vi "Autonomous Independent.vi"() -> ()   [LabVIEW 2023]
doc: "This VI is called when autonomous begins, and will automatically be terminated when autonomous ends. You can carry out timed or sensor driven robot movement independently without needing to return to the caller."
uses:
  <vilib>/Rock Robotics/WPI/ThirdParty/Phoenix-LabVIEW/Motor Controller/Controls/CTRE_Phoenix_MotorControl_ControlMode.ctl
  <vilib>/Rock Robotics/WPI/Utilities/WPI_GetSetVariantRefNum.vi
  <vilib>/Rock Robotics/Network Tables/NT Read String.vi
  <vilib>/Rock Robotics/Network Tables/NT Write Numeric Array.vi
  <vilib>/Rock Robotics/WPI/ThirdParty/Phoenix-LabVIEW/Motor Controller/Get/CTRE_Phoenix_MotorController_GetSelectedSensorData.vi
  <vilib>/Rock Robotics/WPI/ThirdParty/Phoenix-LabVIEW/Pigeon IMU/CTRE_PigeonIMU_GetAccumGyro.vi
  <vilib>/Rock Robotics/WPI/RobotDrive/WPI_RobotDriveArcadeDrive_Standard(NoSaturation).vi
panel:
  out "Limit Switch":bool=TRUE
  out "Y":dbl
  out "X":dbl
  out "Z":dbl
  out "Talon FX LEFT Moter Encoders":i32
  out "Current Movement, for debugging":T1 {"Y Joystick Value" scale=1.0..-1.0; "X Joystick Value" scale=-1.0..1.0}
  in  "Array of robot movements":T2(array[cluster])=[{"X Joystick Value"=0.39393939393939403, "Y Joystick Value"=0.0, "Delay (sec)"=1.0, "Movement Name"="turn"}, {"X Joystick Value"=-0.3737373737373737, "Y Joystick Value"=0.0, "Delay (sec)"=1.0, "Movement Name"="turn back"}] {"Y Joystick Value" scale=1.0..-1.0; "X Joystick Value" scale=-1.0..1.0}
  # "Be sure to right-click and choose Data Operations>>Make Current Value default if you want to save the array values with the VI"
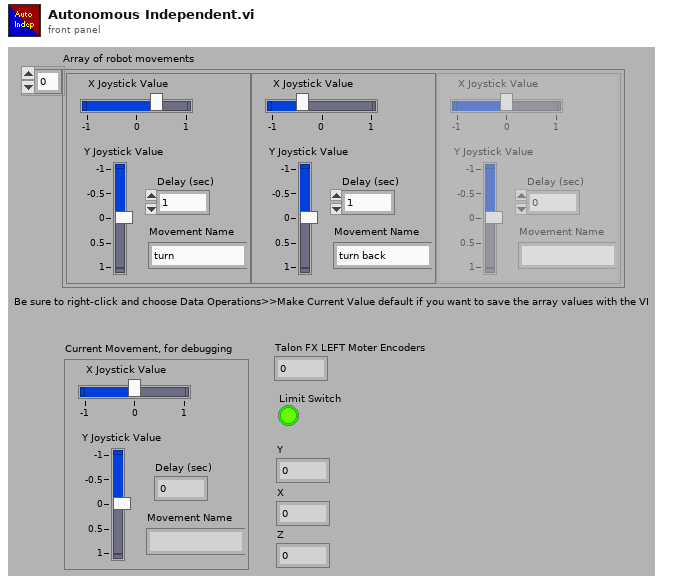
[diagram p1: front panel]
types:
  T1 = cluster{"X Joystick Value":dbl, "Y Joystick Value":dbl, "Delay (sec)":dbl, "Movement Name":string}
  T2 = cluster{"X Joystick Value":dbl, "Y Joystick Value":dbl, "Delay (sec)":dbl, "Movement Name":string}[]
  T3 = typedef "WPI_JoystickDevRef.ctl" = cluster{"Device":T4}
  T4 = typedef "WPI_JoystickDeviceEnum.ctl" = enum16{"USB 0", "USB 1", "USB 2", "USB 3", "USB 4", "USB 5"}
  T5 = typedef "WPI_RobotDriveDevRef.ctl" = cluster{"DevStatus":errorcluster, "Motors[]":T6[], "Square Inputs":bool, "Max Output":dbl}
  T6 = typedef "WPI_MotorControlDeviceRef.ctl" = cluster{"DeviceStatus":errorcluster, "Type":T7, "PWM":cluster{"PWM Channel":T8, "DeadBand":T9}, "CAN":cluster{"Device Number":u8, "SetOutput VI Ref":variant, "GetOutput VI Ref":variant, "Enable VI Ref":variant, "Disable VI Ref":variant, "Data":variant}, "Invert":bool, "DIO PWM":cluster{"PWM \"Enable\" Channel":T8, "DIOChannel":T10, "PWM Rate":dbl}}
  T7 = typedef "WPI_MotorControlType.ctl" = enum16{"PWM", "CAN", "DIO PWM"}
  T8 = typedef "FPGA_DIOPWMChannel.ctl" = enum8{"PWM 0", "PWM 1", "PWM 2", "PWM 3", "PWM 4", "PWM 5", "PWM 6", "PWM 7", "PWM 8", "PWM 9", "PWM MXP 0", "PWM MXP 1", "PWM MXP 2", "PWM MXP 3", "PWM MXP 4", "PWM MXP 5", "PWM MXP 6", "PWM MXP 7", "PWM MXP 8", "PWM MXP 9", "Invalid"}
  T9 = typedef "WPI_PWMDeadband.ctl" = cluster{"Name":string, "maxPositivePwm":i32, "minPositivePwm":i32, "centerPwm":i32, "maxNegativePwm":i32, "minNegativePwm":i32, "angularRange":u16}
  T10 = typedef "FPGA_DIOChannel.ctl" = enum8{"DIO 0", "DIO 1", "DIO 2", "DIO 3", "DIO 4", "DIO 5", "DIO 6", "DIO 7", "DIO 8", "DIO 9", "DIO MXP 0", "DIO MXP 1", "DIO MXP 2", "DIO MXP 3", "DIO MXP 4", "DIO MXP 5", "DIO MXP 6", "DIO MXP 7", "DIO MXP 8", "DIO MXP 9", "DIO MXP 10", "DIO MXP 11", "DIO MXP 12", "DIO MXP 13", "DIO MXP 14", "DIO MXP 15", "SPI Port CS1", "SPI Port CS2", "SPI Port CS3", "SPI Port MISO", "SPI Port MOSI", "Invalid"}
  T11 = typedef "CTRE_Phoenix_MotorControl_ControlMode.ctl" = u16
  T12 = typedef "CTRE_PigeonIMU_DeviceRef.ctl" = cluster{"DeviceStatus":errorcluster, "Device Number":u8, "Type":T13, "Device ID":u32, "Handle":u64, "UsageFrame":u32, "Library Path":path}
  T13 = typedef "CTRE_PigeonIMU_ConnectionType.ctl" = u32
  T14 = typedef "WPI_SwitchDevRef.ctl" = cluster{"DevStatus":errorcluster, "DIO Channel":T10, "CntIndex":T15, "Normally Closed":bool}
  T15 = typedef "FPGA_CounterCtrSystemIndex.ctl" = enum8{"Ctr 0", "Ctr 1", "Ctr 2", "Ctr 3", "Ctr 4", "Ctr 5", "Ctr 6", "Ctr 7", "Invalid"}
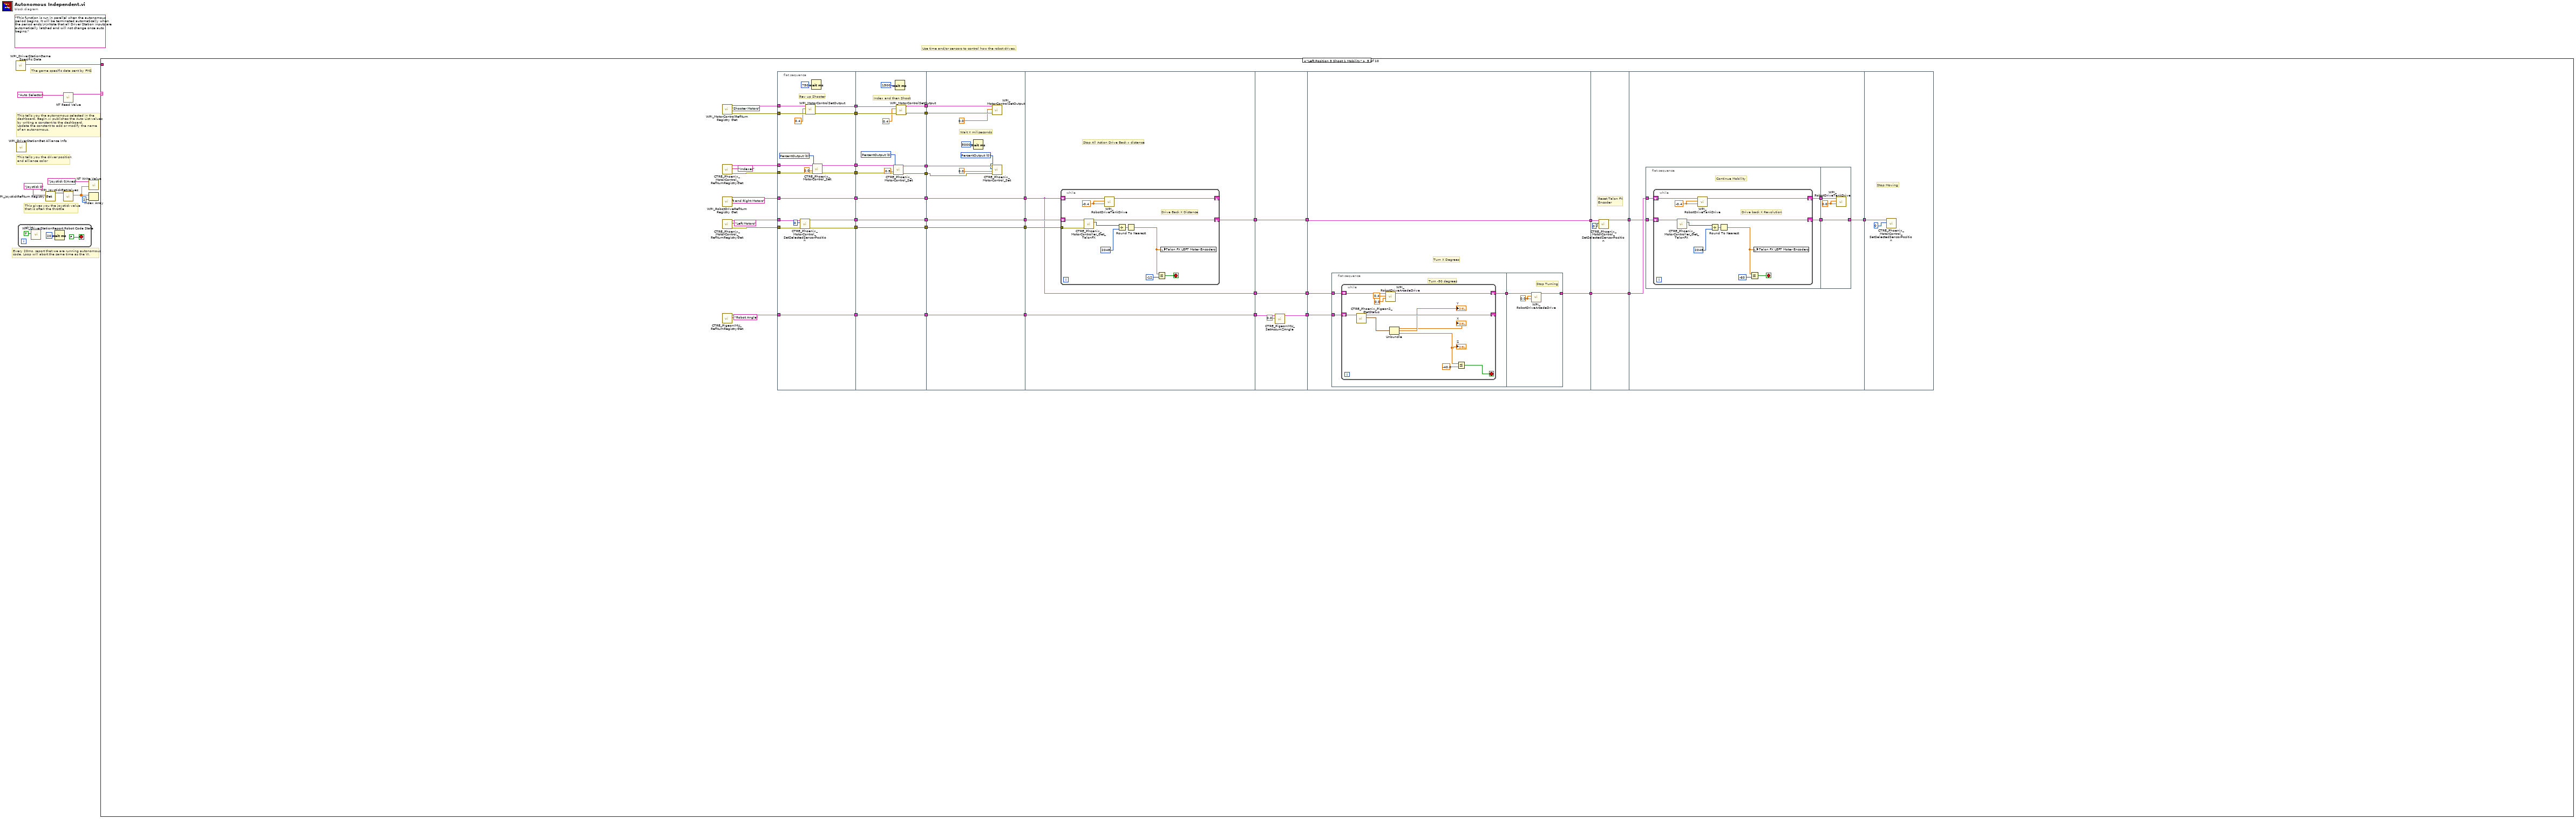
[diagram p0: block diagram]
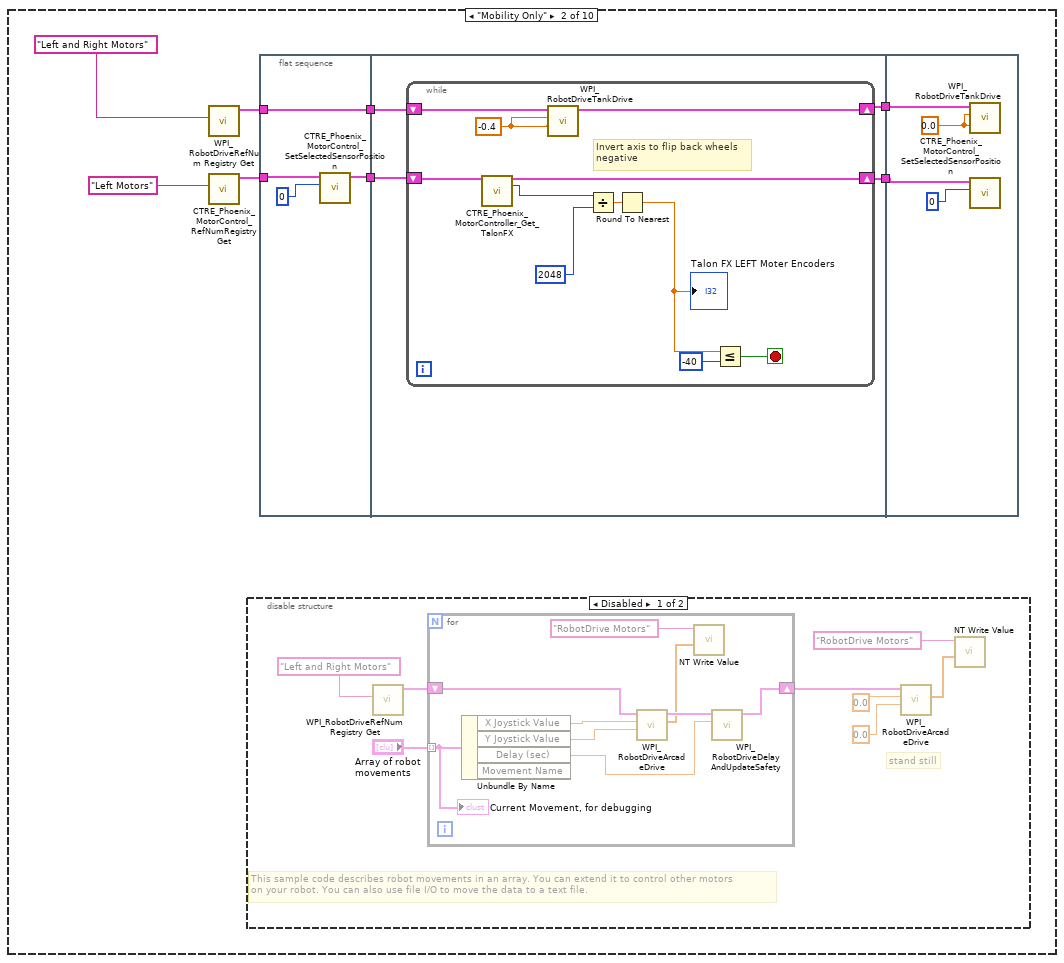
[diagram p3: hidden frame]
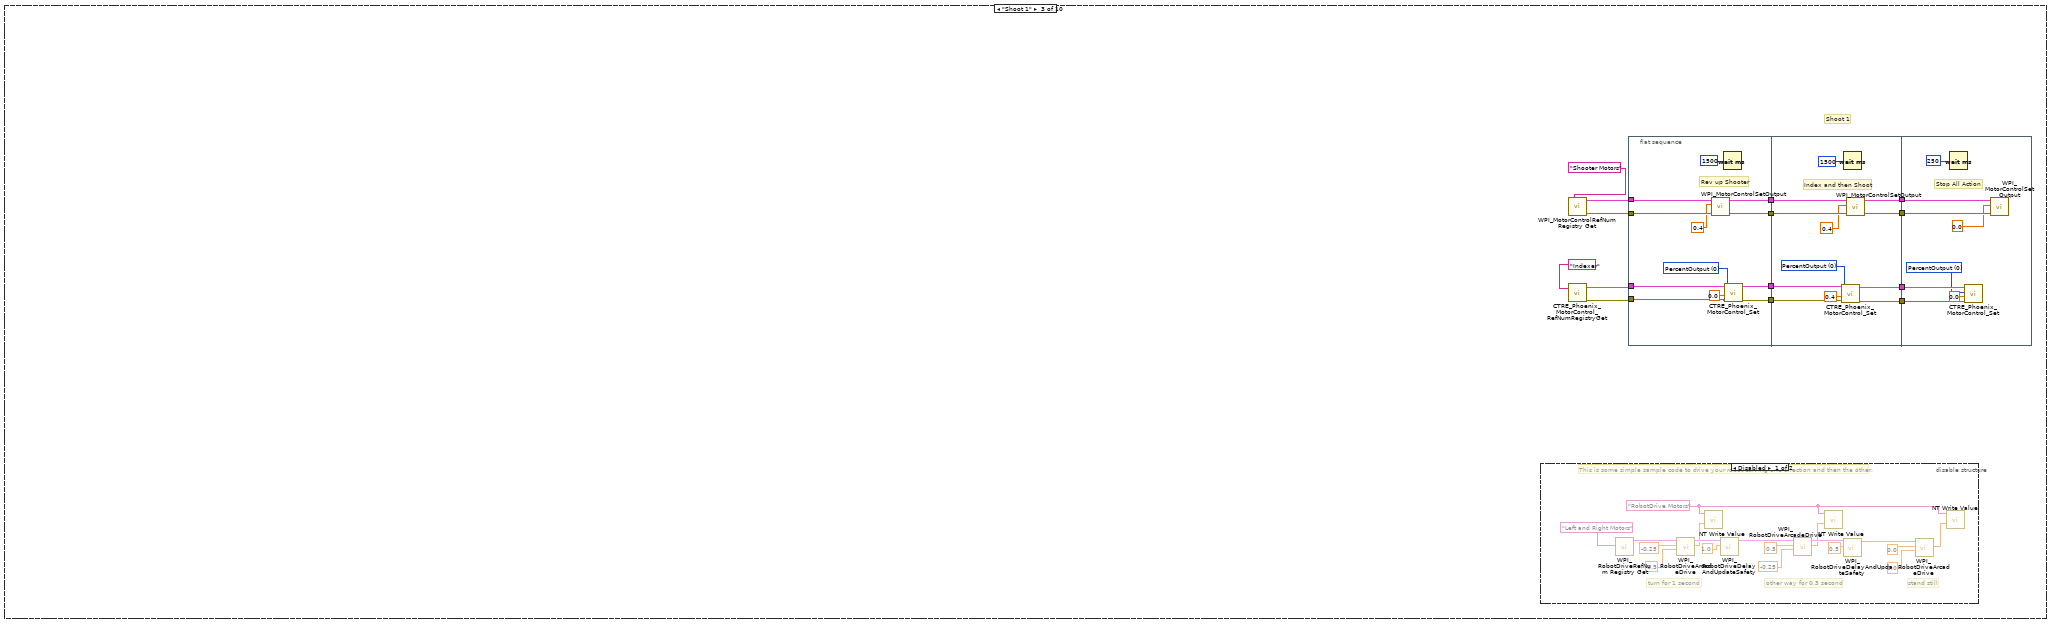
[diagram p5: hidden frame]
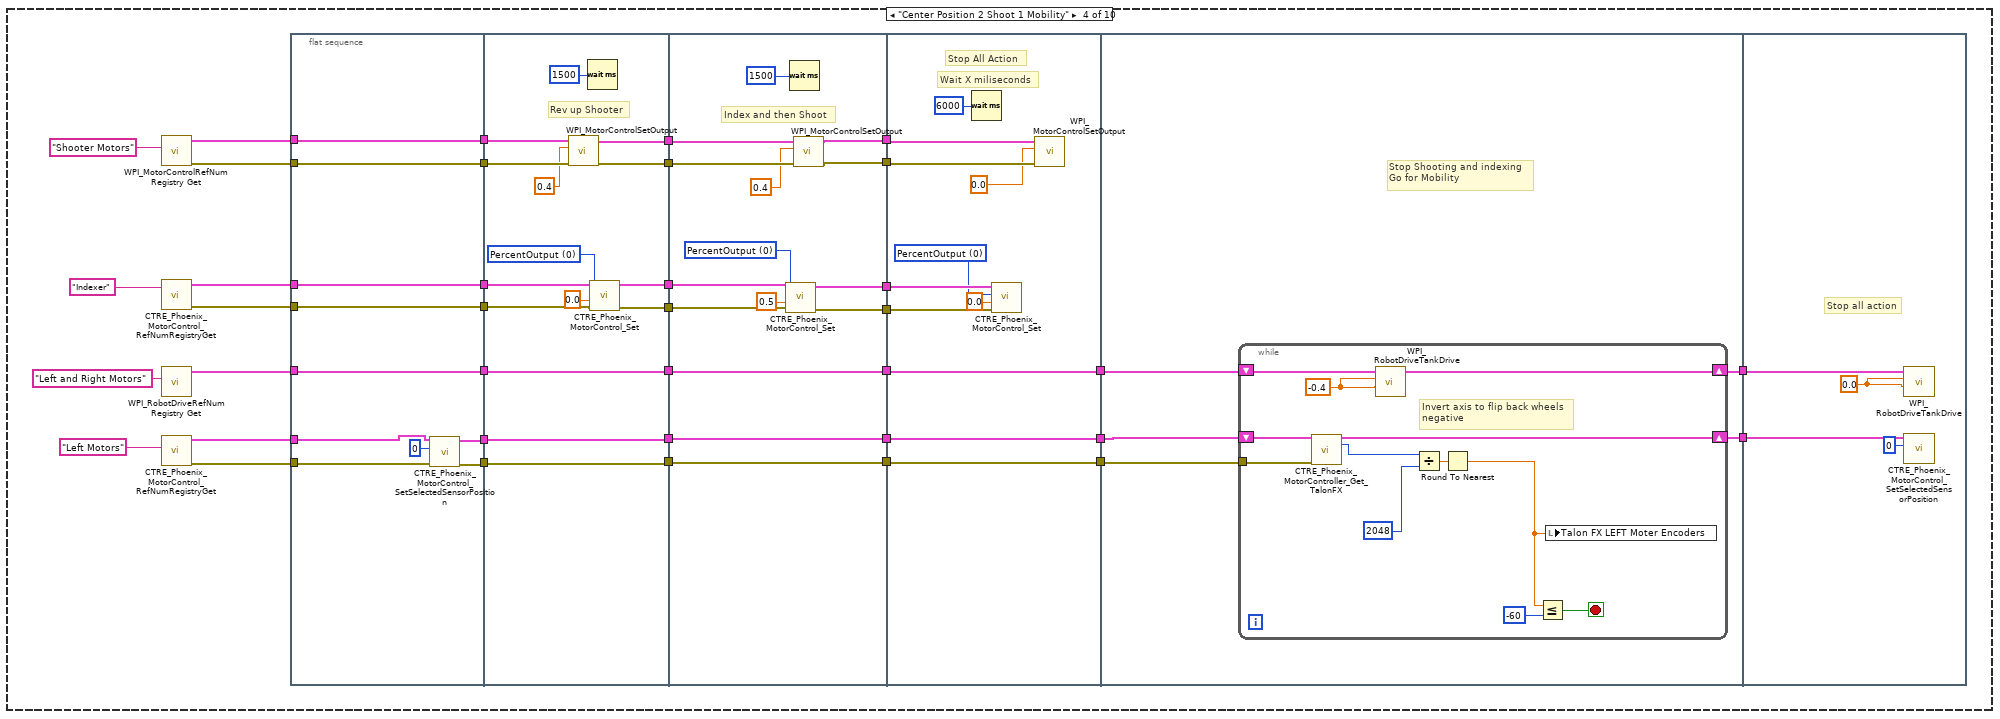
[diagram p7: hidden frame]
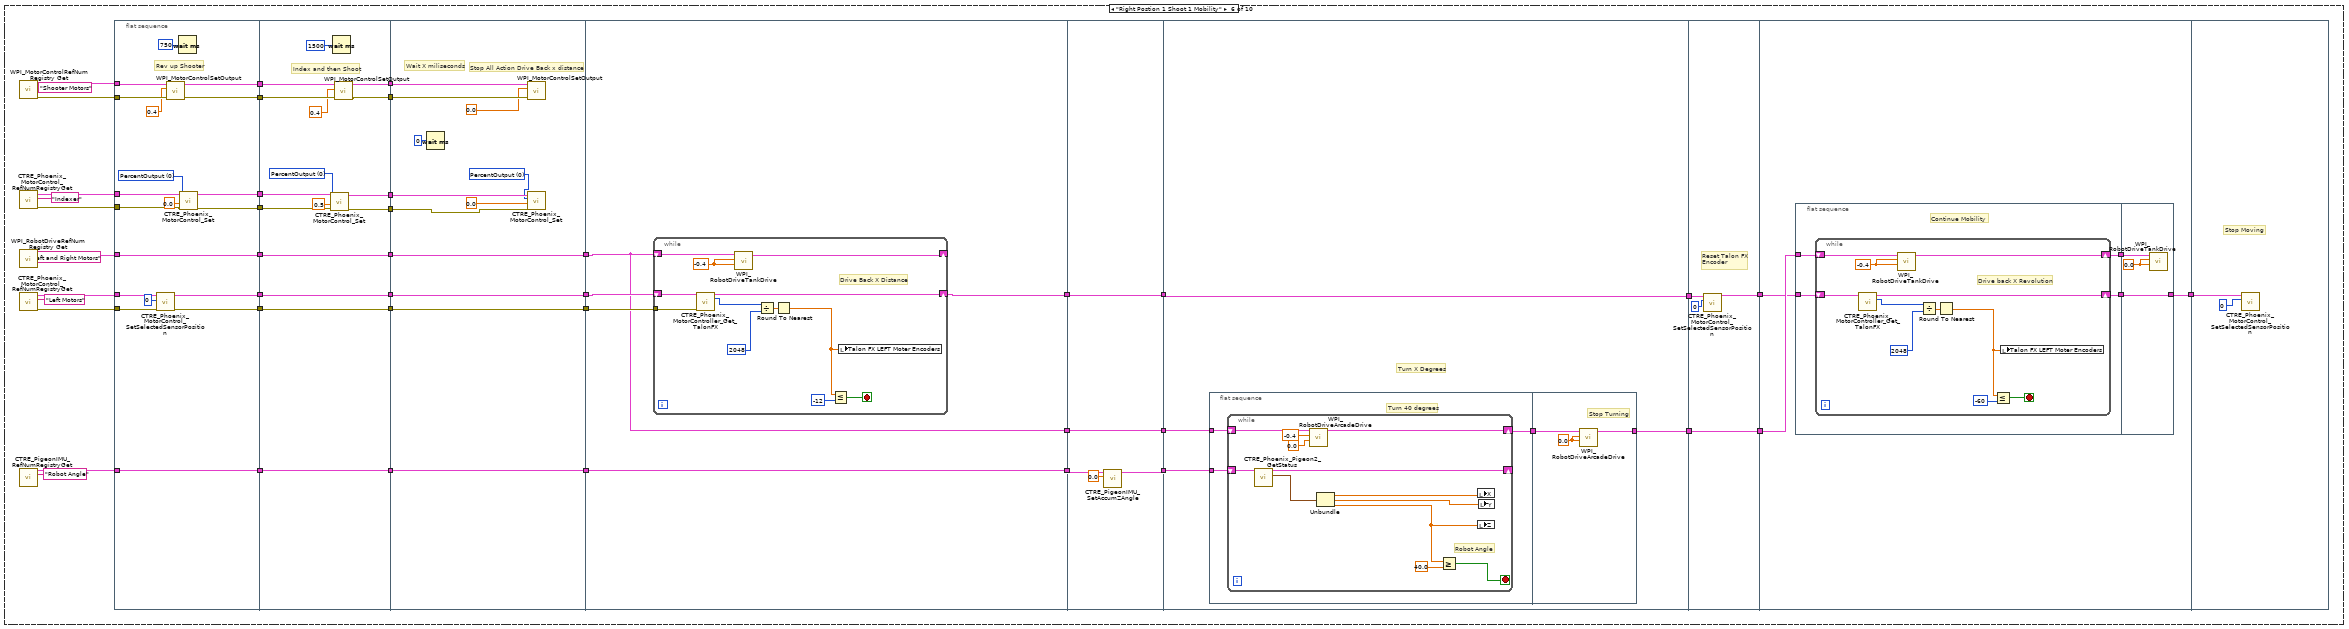
[diagram p8: hidden frame]
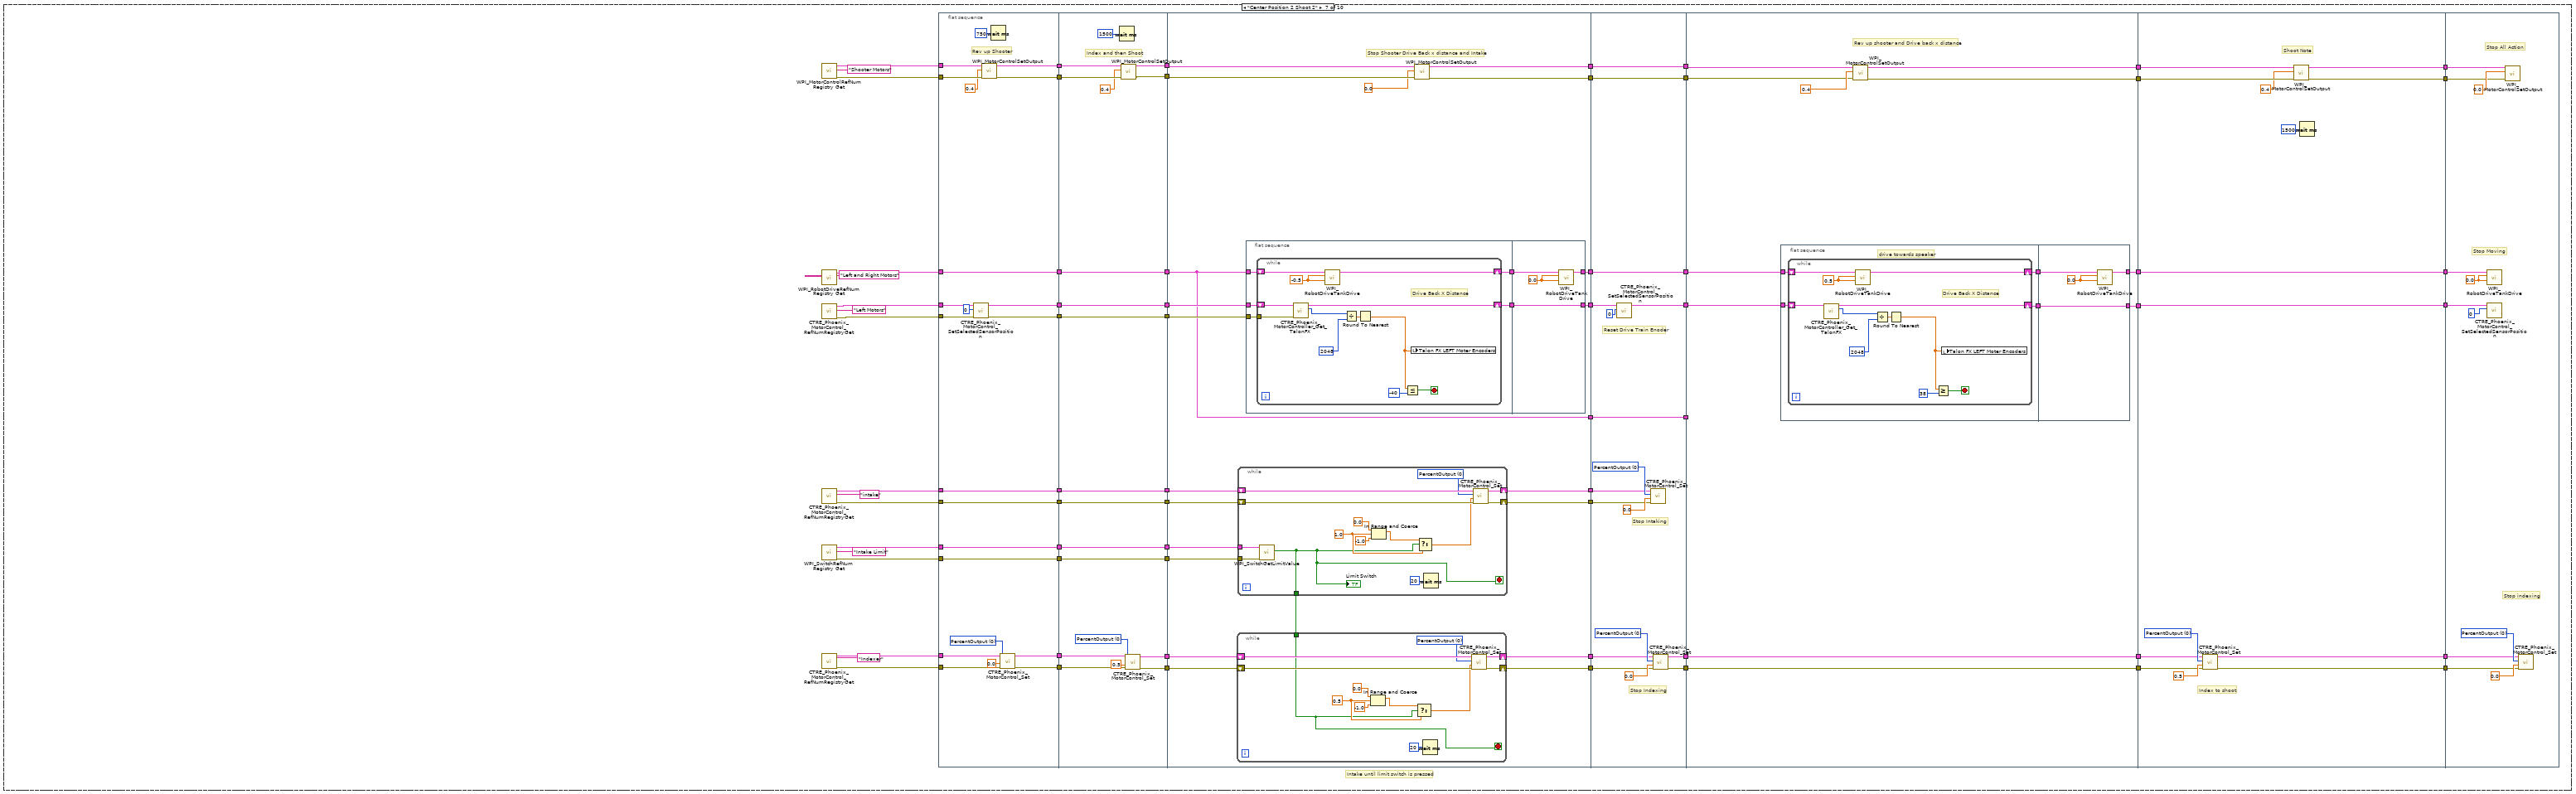
[diagram p9: hidden frame]
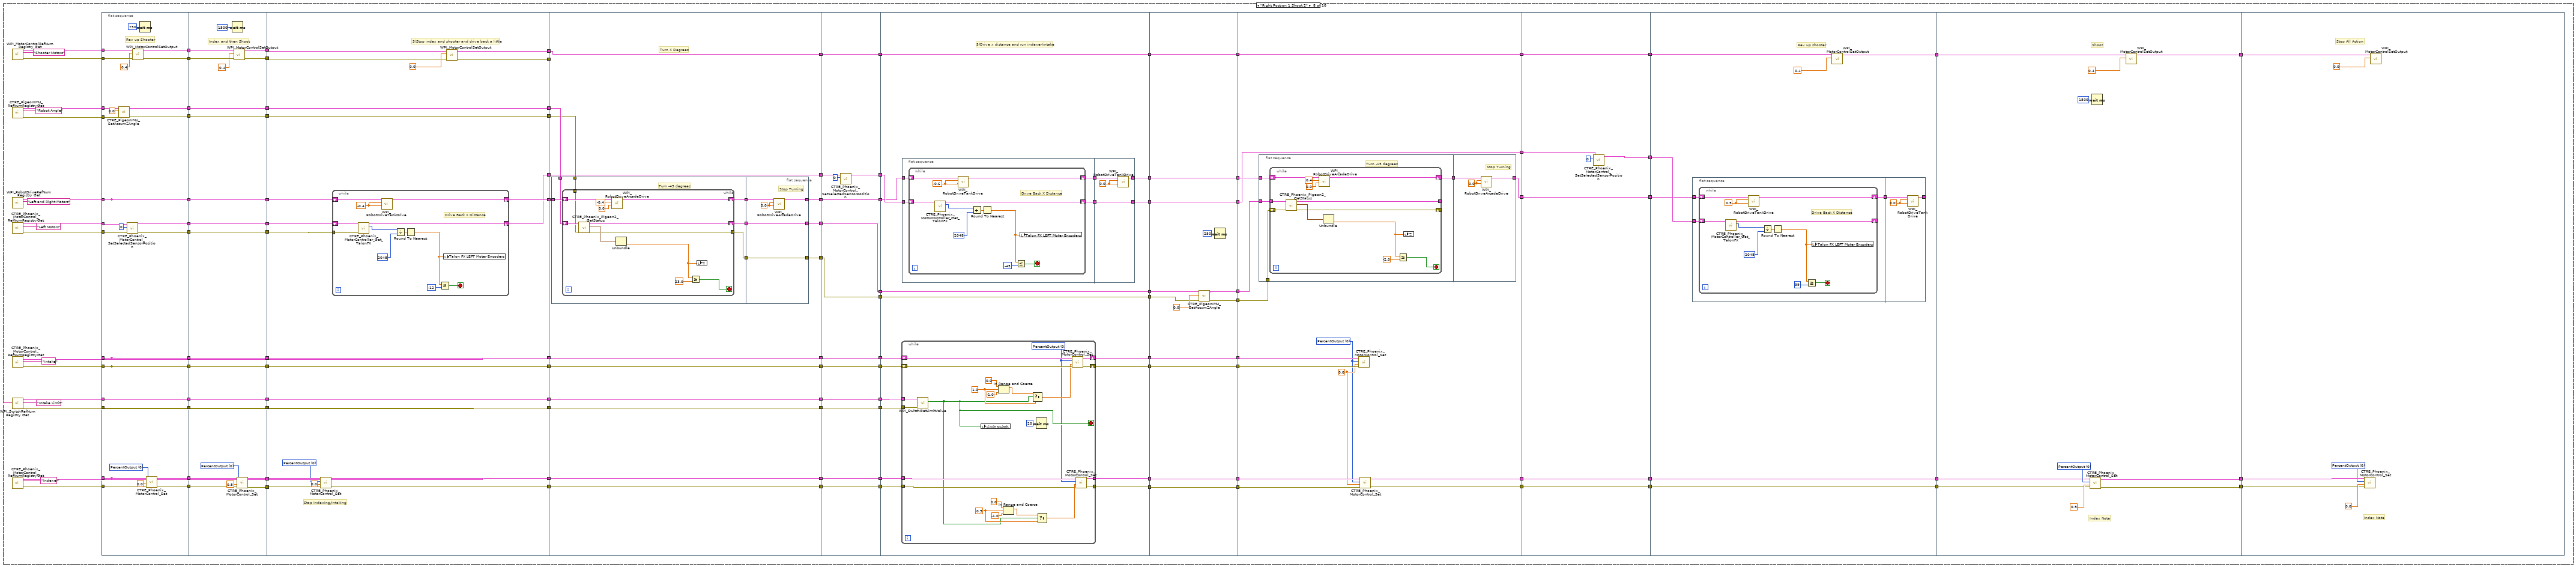
[diagram p10: hidden frame]
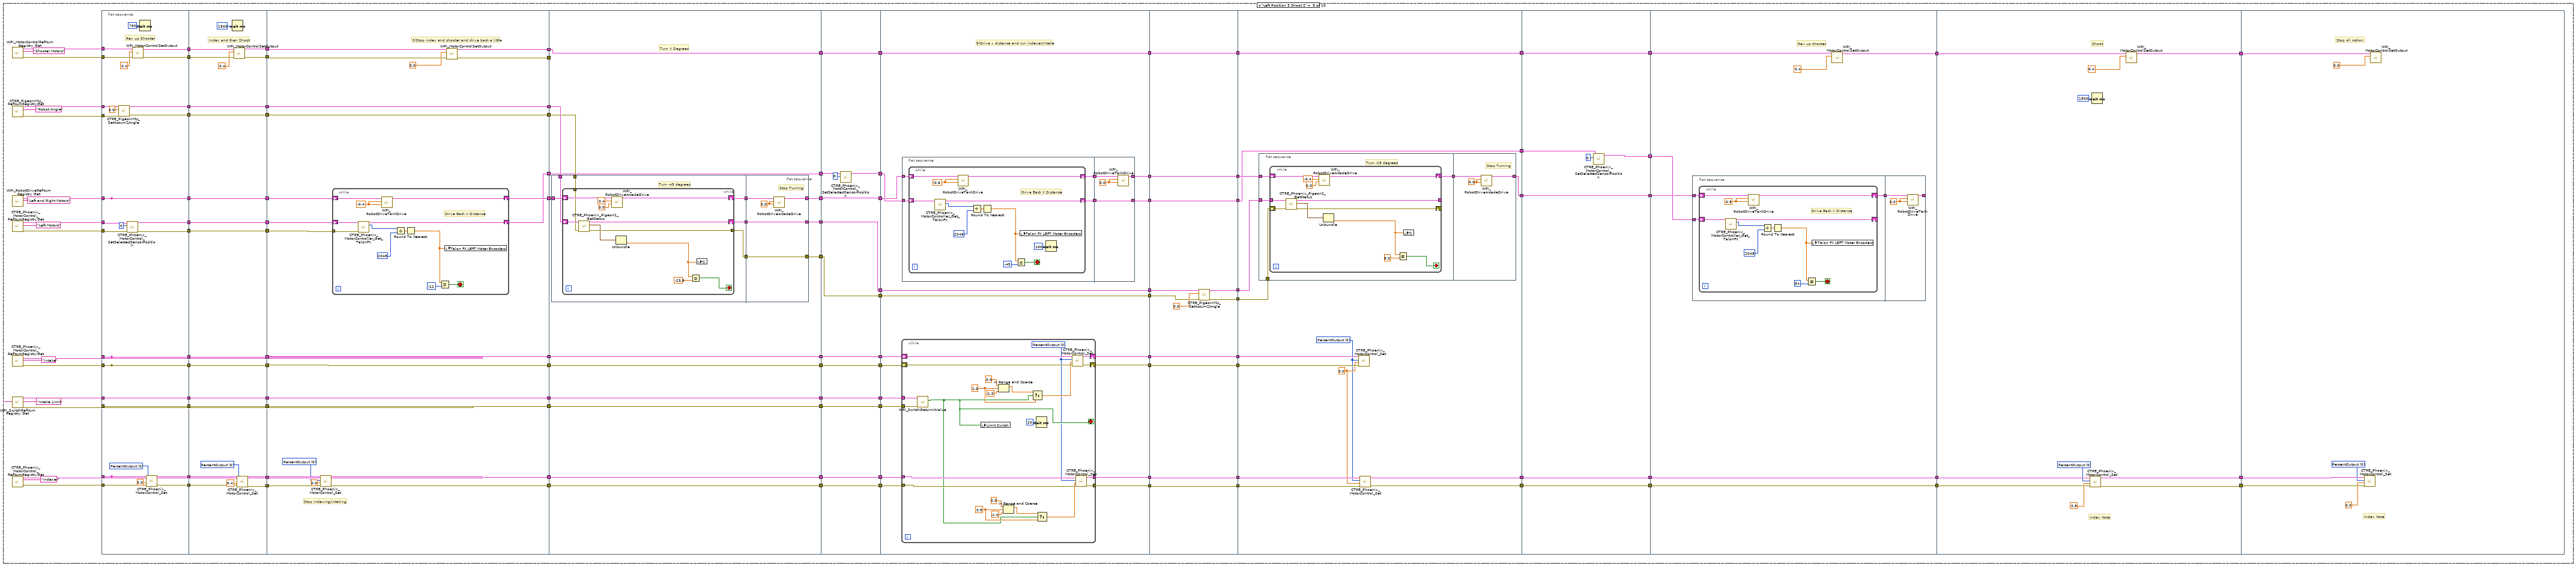
[diagram p11: hidden frame]
diagram:
  (unwired) "This function is run in parallel when the autonomous period begins. It will be terminated automatically when the period ends.\n\nNote that all Driver Station inputs are automatically latched and will not change once auto begins."
  # "The game specific data sent by FMS"
  # "This tells you the autonomous selected in the \ndashboard. Begin.vi publishes the Auto List values\nby writing a constant to the dashboard.\nUpdate the constant to add or modify the name\nof an autonomous."
  # "Every 20ms, report that we are running autonomous\ncode. Loop will abort the same time as the VI."
  # "This gives you the joystick value\nthat is often the throttle"
  # "Use time and/or sensors to control how the robot drives."
  # "This tells you the driver position\nand alliance color"
  n1 = call <vilib>:"WPI_DriverStationGame Specific Data.vi"() -> ("Game Specific Data"=w1:string)  [unwired: 11 in]
  n2 = call <vilib>:"WPI_DriverStationGet Alliance Info.vi"() -> ()  [unwired: 12 out]
  n3 = while {
    stop <- FALSE stop-if-true
    n4 = call <vilib>:"WPI_DriverStationReport Robot Code State.vi"("Autonomous"=TRUE) -> ()  [unwired: 10 in, 1 out]
    n5 = Wait (ms)(milliseconds to wait=u32 20) -> ()  [unwired: 1 out]
  }
  n6 = call <vilib>:"WPI_JoystickRefNum Registry Get.vi"("refnum name"="Joystick 0") -> ("JoystickDevRef"=w7:T3)  [unwired: 1 in, 9 out]
  n7 = call <vilib>:"WPI_JoystickGetValues.vi"("JoystickDevRef"=w7) -> ("Axes"=w3:dbl[])  [unwired: 6 in, 4 out]
  n8 = call-poly <vilib>:"NT Read Value.vi"("name"="Auto Selector" ("Name")) -> ("value"=w4:string)  [unwired: 8 in, 2 out]
  n9 = call-poly <vilib>:"NT Write Value.vi"("value"=w3, "name"="Joystick 0/Axes" ("Name")) -> ()  [unwired: 9 in, 1 out]
  n10 = Index Array(array=w3, index=2) -> ()  [unwired: 1 out]
  n11 = case shown="\"Left Position 3 Shoot 1 Mobility\"" w4 {
    tunnel: w1 -> [_ _ _ _ _ _ _ _ _ _]
    frame Default {
      # "You can put your main auto here, or you can right-click on the case and make any\nother frame be the default case."
      # "This is the frame that will execute if no selection is made, or if it is not recognized"
    }
    frame "Mobility Only" {
      n12 = call <vilib>:"WPI_RobotDriveRefNum Registry Get.vi"("refnum name"="Left and Right Motors") -> ("RobotDriveDevRef"=w17:T5)  [unwired: 9 in, 1 out]
      n13 = call <vilib>:"CTRE_Phoenix_MotorControl_RefNumRegistryGet.vi"("refnum name"="Left Motors") -> ("PhoenixMotorControlDevRef"=w16:T6)  [unwired: 9 in, 1 out]
      n14 = disable-structure shown="Disabled" {
        frame Disabled {
          # "stand still"
          # "This sample code describes robot movements in an array. You can extend it to control other motors\non your robot. You can also use file I/O to move the data to a text file."
          n15 = call <vilib>:"WPI_RobotDriveRefNum Registry Get.vi"("refnum name"="Left and Right Motors") -> ("RobotDriveDevRef"=w49:T5)  [unwired: 1 in, 9 out]
          n16 = for {
            shift-right: [w57] -> w44
            shift-left: w49 -> [w58]
            tunnel: "Array of robot movements" -> [w53] mode=indexing
            n17 = Unbundle By Name(w53) -> ("X Joystick Value"=w56:dbl, "Y Joystick Value"=w55:dbl, "Delay (sec)"=w54:dbl)  [unwired: 1 out]
            n18 = call-poly <vilib>:"WPI_RobotDriveArcadeDrive.vi"("Y axis value"=w55, "X axis value"=w56, "RobotDriveDevRef"=w58) -> ("Motor Values"=w51:dbl[], "RobotDriveDevRef"=w59:T5)  [unwired: 1 in, 6 out]
            n19 = call-poly <vilib>:"NT Write Value.vi"("value"=w51, "name"="RobotDrive Motors" ("Name")) -> ()  [unwired: 9 in, 1 out]
            n20 = call <vilib>:"WPI_RobotDriveDelayAndUpdateSafety.vi"("Delay (s)"=w54, "RobotDriveDevRef"=w59) -> ("RobotDriveDevRef 2"=w57:T5)  [unwired: 8 in, 1 out]
            "Current Movement, for debugging" <- w53
          }
          n21 = call-poly <vilib>:"WPI_RobotDriveArcadeDrive.vi"("Y axis value"=0.0 ("X axis value"), "X axis value"=0.0, "RobotDriveDevRef"=w44) -> ("Motor Values"=w47:dbl[])  [unwired: 1 in, 7 out]
          n22 = call-poly <vilib>:"NT Write Value.vi"("value"=w47, "name"="RobotDrive Motors" ("Name")) -> ()  [unwired: 9 in, 1 out]
        }
        frame Enabled {
        }
      }
      n23 = flat-sequence {
        tunnel: w16 -> [w21]
        tunnel: w17 -> [w23]
        tunnel: [w23] -> w13
        tunnel: [w20] -> w12
        tunnel: [w26] -> w19
        tunnel: [w25] -> w18
        tunnel: w13 -> [w27]
        tunnel: w12 -> [w24]
        tunnel: w19 -> [w41]
        tunnel: w18 -> [w40]
        frame #0 {
          n24 = call <vilib>:"CTRE_Phoenix_MotorControl_SetSelectedSensorPosition.vi"("New Sensor Position"=0, "PhoenixMotorControlDevRef"=w21) -> ("PhoenixMotorControlDevRef"=w20:T6)  [unwired: 8 in, 1 out]
        }
        frame #1 {
          n25 = while {
            shift-right: [w36] -> w26
            shift-left: w27 -> [w38]
            shift-right: [w35] -> w25
            shift-left: w24 -> [w37]
            stop <- w34 stop-if-true
            w33 = -0.4 ("Left axis value")
            # "Invert axis to flip back wheels\nnegative"
            n26 = call-poly <vilib>:"CTRE_Phoenix_MotorController_Get_TalonFX.vi"("PhoenixMotorControlDevRef"=w37) -> ("PhoenixMotorControlDevRef"=w35:T6, "Position (Raw Sensor Units)"=w29:i32)  [unwired: 11 in, 2 out]
            n27 = call <vilib>:"WPI_RobotDriveTankDrive.vi"("Right axis value"=w33, "Left axis value"=w33, "RobotDriveDevRef"=w38) -> ("RobotDriveDevRef"=w36:T5)  [unwired: 6 in, 2 out]
            n28 = Divide(x=w29, y=2048) -> (x/y=w30:dbl)
            n29 = Round To Nearest(number=w30) -> (nearest integer value=w28:dbl)
            "Talon FX LEFT Moter Encoders" <- w28
            n30 = Less Or Equal?(x=w28, y=-40) -> (x <= y?=w34:bool)
          }
        }
        frame #2 {
          w42 = 0.0
          n31 = call <vilib>:"WPI_RobotDriveTankDrive.vi"("Right axis value"=w42, "Left axis value"=w42, "RobotDriveDevRef"=w41) -> ()  [unwired: 6 in, 3 out]
          n32 = call <vilib>:"CTRE_Phoenix_MotorControl_SetSelectedSensorPosition.vi"("New Sensor Position"=0, "PhoenixMotorControlDevRef"=w40) -> ()  [unwired: 8 in, 2 out]
        }
      }
    }
    frame "Shoot 1" {
      # "Shoot 1"
      n33 = disable-structure shown="Disabled" {
        frame Disabled {
          w107 = "RobotDrive Motors" ("Name")
          # "This is some simple sample code to drive your robot curving one direction and then the other."
          # "stand still"
          # "other way for 0.5 second"
          # "turn for 1 second"
          n34 = call <vilib>:"WPI_RobotDriveRefNum Registry Get.vi"("refnum name"="Left and Right Motors") -> ("RobotDriveDevRef"=w123:T5)  [unwired: 1 in, 9 out]
          n35 = call-poly <vilib>:"WPI_RobotDriveArcadeDrive.vi"("Y axis value"=0.5 ("X axis value"), "X axis value"=-0.25, "RobotDriveDevRef"=w123) -> ("Motor Values"=w106:dbl[], "RobotDriveDevRef"=w116:T5)  [unwired: 1 in, 6 out]
          n36 = call-poly <vilib>:"NT Write Value.vi"("value"=w106, "name"=w107) -> ()  [unwired: 9 in, 1 out]
          n37 = call <vilib>:"WPI_RobotDriveDelayAndUpdateSafety.vi"("Delay (s)"=1.0, "RobotDriveDevRef"=w116) -> ("RobotDriveDevRef 2"=w117:T5)  [unwired: 8 in, 1 out]
          n38 = call-poly <vilib>:"WPI_RobotDriveArcadeDrive.vi"("Y axis value"=-0.25 ("X axis value"), "X axis value"=0.5, "RobotDriveDevRef"=w117) -> ("Motor Values"=w108:dbl[], "RobotDriveDevRef"=w118:T5)  [unwired: 1 in, 6 out]
          n39 = call-poly <vilib>:"NT Write Value.vi"("value"=w108, "name"=w107) -> ()  [unwired: 9 in, 1 out]
          n40 = call <vilib>:"WPI_RobotDriveDelayAndUpdateSafety.vi"("Delay (s)"=0.5, "RobotDriveDevRef"=w118) -> ("RobotDriveDevRef 2"=w119:T5)  [unwired: 8 in, 1 out]
          n41 = call-poly <vilib>:"WPI_RobotDriveArcadeDrive.vi"("Y axis value"=0.0 ("X axis value"), "X axis value"=0.0, "RobotDriveDevRef"=w119) -> ("Motor Values"=w109:dbl[])  [unwired: 1 in, 7 out]
          n42 = call-poly <vilib>:"NT Write Value.vi"("value"=w109, "name"=w107) -> ()  [unwired: 9 in, 1 out]
        }
        frame Enabled {
        }
      }
      n43 = call <vilib>:"WPI_MotorControlRefNum Registry Get.vi"("refnum name"="Shooter Motors") -> ("error out"=w62:errorcluster, "MotorControlDevRef"=w63:T6)  [unwired: 9 in]
      n44 = call <vilib>:"CTRE_Phoenix_MotorControl_RefNumRegistryGet.vi"("refnum name"="Indexer") -> ("error out"=w64:errorcluster, "PhoenixMotorControlDevRef"=w65:T6)  [unwired: 9 in]
      n45 = flat-sequence {
        tunnel: w63 -> [w85]
        tunnel: w62 -> [w84]
        tunnel: [w81] -> w73
        tunnel: [w80] -> w72
        tunnel: [w79] -> w71
        tunnel: [w78] -> w70
        tunnel: w65 -> [w77]
        tunnel: w64 -> [w76]
        tunnel: w73 -> [w96]
        tunnel: w72 -> [w95]
        tunnel: [w94] -> w69
        tunnel: [w93] -> w68
        tunnel: [w91] -> w67
        tunnel: [w90] -> w66
        tunnel: w71 -> [w89]
        tunnel: w70 -> [w88]
        tunnel: w69 -> [w105]
        tunnel: w68 -> [w104]
        tunnel: w67 -> [w101]
        tunnel: w66 -> [w100]
        frame #0 {
          w74 = T11 0 items=["PercentOutput"=0, "Position"=1, "Velocity"=2, "Current"=3, "Follower"=5, "MotionProfile"=6, "MotionMagic"=7, "MotionProfileArc"=10, "Disabled"=15] ("Control Mode")
          # "Rev up Shooter"
          n46 = call <vilib>:"WPI_MotorControlSetOutput.vi"("error in (no error)"=w84, "Output"=0.4, "MotorControlDevRef"=w85) -> ("error out"=w80:errorcluster, "MotorControlDevRef"=w81:T6)  [unwired: 6 in, 1 out]
          n47 = Wait (ms)(milliseconds to wait=u32 1500) -> ()  [unwired: 1 out]
          n48 = call <vilib>:"CTRE_Phoenix_MotorControl_Set.vi"("error in (no error)"=w76, "Output"=0.0, "Control Mode"=w74, "PhoenixMotorControlDevRef"=w77) -> ("error out"=w78:errorcluster, "PhoenixMotorControlDevRef"=w79:T6)  [unwired: 6 in]
        }
        frame #1 {
          w86 = T11 0 items=["PercentOutput"=0, "Position"=1, "Velocity"=2, "Current"=3, "Follower"=5, "MotionProfile"=6, "MotionMagic"=7, "MotionProfileArc"=10, "Disabled"=15] ("Control Mode")
          # "Index and then Shoot"
          n49 = call <vilib>:"CTRE_Phoenix_MotorControl_Set.vi"("error in (no error)"=w88, "Output"=0.4, "Control Mode"=w86, "PhoenixMotorControlDevRef"=w89) -> ("error out"=w90:errorcluster, "PhoenixMotorControlDevRef"=w91:T6)  [unwired: 6 in]
          n50 = Wait (ms)(milliseconds to wait=u32 1500) -> ()  [unwired: 1 out]
          n51 = call <vilib>:"WPI_MotorControlSetOutput.vi"("error in (no error)"=w95, "Output"=0.4, "MotorControlDevRef"=w96) -> ("error out"=w93:errorcluster, "MotorControlDevRef"=w94:T6)  [unwired: 6 in, 1 out]
        }
        frame #2 {
          w98 = T11 0 items=["PercentOutput"=0, "Position"=1, "Velocity"=2, "Current"=3, "Follower"=5, "MotionProfile"=6, "MotionMagic"=7, "MotionProfileArc"=10, "Disabled"=15] ("Control Mode")
          # "Stop All Action"
          n52 = Wait (ms)(milliseconds to wait=u32 250) -> ()  [unwired: 1 out]
          n53 = call <vilib>:"CTRE_Phoenix_MotorControl_Set.vi"("error in (no error)"=w100, "Output"=0.0, "Control Mode"=w98, "PhoenixMotorControlDevRef"=w101) -> ()  [unwired: 6 in, 2 out]
          n54 = call <vilib>:"WPI_MotorControlSetOutput.vi"("error in (no error)"=w104, "Output"=0.0, "MotorControlDevRef"=w105) -> ()  [unwired: 6 in, 3 out]
        }
      }
    }
    frame "Center Position 2 Shoot 1 Mobility" {
      n55 = call <vilib>:"WPI_MotorControlRefNum Registry Get.vi"("refnum name"="Shooter Motors") -> ("error out"=w138:errorcluster, "MotorControlDevRef"=w139:T6)  [unwired: 9 in]
      n56 = call <vilib>:"CTRE_Phoenix_MotorControl_RefNumRegistryGet.vi"("refnum name"="Indexer") -> ("error out"=w140:errorcluster, "PhoenixMotorControlDevRef"=w141:T6)  [unwired: 9 in]
      n57 = call <vilib>:"WPI_RobotDriveRefNum Registry Get.vi"("refnum name"="Left and Right Motors") -> ("RobotDriveDevRef"=w133:T5)  [unwired: 9 in, 1 out]
      n58 = call <vilib>:"CTRE_Phoenix_MotorControl_RefNumRegistryGet.vi"("refnum name"="Left Motors") -> ("error out"=w131:errorcluster, "PhoenixMotorControlDevRef"=w132:T6)  [unwired: 9 in]
      n59 = flat-sequence {
        tunnel: w131 -> [w163]
        tunnel: w132 -> [w164]
        tunnel: w133 -> [w166]
        tunnel: w140 -> [w167]
        tunnel: w141 -> [w168]
        tunnel: w138 -> [w169]
        tunnel: w139 -> [w170]
        tunnel: [w170] -> w130
        tunnel: [w169] -> w129
        tunnel: [w168] -> w128
        tunnel: [w167] -> w127
        tunnel: [w166] -> w126
        tunnel: [w161] -> w125
        tunnel: [w162] -> w124
        tunnel: [w181] -> w160
        tunnel: [w180] -> w159
        tunnel: [w179] -> w158
        tunnel: [w178] -> w157
        tunnel: [w173] -> w156
        tunnel: [w172] -> w155
        tunnel: [w171] -> w154
        tunnel: w130 -> [w185]
        tunnel: w129 -> [w184]
        tunnel: w128 -> [w177]
        tunnel: w127 -> [w176]
        tunnel: w126 -> [w173]
        tunnel: w125 -> [w172]
        tunnel: w124 -> [w171]
        tunnel: w160 -> [w199]
        tunnel: w159 -> [w198]
        tunnel: [w197] -> w153
        tunnel: [w196] -> w152
        tunnel: [w194] -> w151
        tunnel: [w193] -> w150
        tunnel: w158 -> [w192]
        tunnel: w157 -> [w191]
        tunnel: w156 -> [w188]
        tunnel: [w188] -> w149
        tunnel: w155 -> [w187]
        tunnel: [w187] -> w148
        tunnel: w154 -> [w186]
        tunnel: [w186] -> w147
        tunnel: w153 -> [w211]
        tunnel: w152 -> [w210]
        tunnel: w151 -> [w208]
        tunnel: w150 -> [w207]
        tunnel: w149 -> [w204]
        tunnel: [w204] -> w146
        tunnel: w148 -> [w203]
        tunnel: [w203] -> w145
        tunnel: [w202] -> w144
        tunnel: w147 -> [w202]
        tunnel: w146 -> [w216]
        tunnel: w145 -> [w215]
        tunnel: w144 -> [w214]
        tunnel: [w213] -> w143
        tunnel: [w212] -> w142
        tunnel: w143 -> [w231]
        tunnel: w142 -> [w230]
        frame #0 {
          n60 = call <vilib>:"CTRE_Phoenix_MotorControl_SetSelectedSensorPosition.vi"("error in (no error)"=w163, "New Sensor Position"=0, "PhoenixMotorControlDevRef"=w164) -> ("error out"=w162:errorcluster, "PhoenixMotorControlDevRef"=w161:T6)  [unwired: 7 in]
        }
        frame #1 {
          w174 = T11 0 items=["PercentOutput"=0, "Position"=1, "Velocity"=2, "Current"=3, "Follower"=5, "MotionProfile"=6, "MotionMagic"=7, "MotionProfileArc"=10, "Disabled"=15] ("Control Mode")
          # "Rev up Shooter"
          n61 = call <vilib>:"WPI_MotorControlSetOutput.vi"("error in (no error)"=w184, "Output"=0.4, "MotorControlDevRef"=w185) -> ("error out"=w180:errorcluster, "MotorControlDevRef"=w181:T6)  [unwired: 6 in, 1 out]
          n62 = Wait (ms)(milliseconds to wait=u32 1500) -> ()  [unwired: 1 out]
          n63 = call <vilib>:"CTRE_Phoenix_MotorControl_Set.vi"("error in (no error)"=w176, "Output"=0.0, "Control Mode"=w174, "PhoenixMotorControlDevRef"=w177) -> ("error out"=w178:errorcluster, "PhoenixMotorControlDevRef"=w179:T6)  [unwired: 6 in]
        }
        frame #2 {
          w189 = T11 0 items=["PercentOutput"=0, "Position"=1, "Velocity"=2, "Current"=3, "Follower"=5, "MotionProfile"=6, "MotionMagic"=7, "MotionProfileArc"=10, "Disabled"=15] ("Control Mode")
          # "Index and then Shoot"
          n64 = call <vilib>:"CTRE_Phoenix_MotorControl_Set.vi"("error in (no error)"=w191, "Output"=0.5, "Control Mode"=w189, "PhoenixMotorControlDevRef"=w192) -> ("error out"=w193:errorcluster, "PhoenixMotorControlDevRef"=w194:T6)  [unwired: 6 in]
          n65 = Wait (ms)(milliseconds to wait=u32 1500) -> ()  [unwired: 1 out]
          n66 = call <vilib>:"WPI_MotorControlSetOutput.vi"("error in (no error)"=w198, "Output"=0.4, "MotorControlDevRef"=w199) -> ("error out"=w196:errorcluster, "MotorControlDevRef"=w197:T6)  [unwired: 6 in, 1 out]
        }
        frame #3 {
          w205 = T11 0 items=["PercentOutput"=0, "Position"=1, "Velocity"=2, "Current"=3, "Follower"=5, "MotionProfile"=6, "MotionMagic"=7, "MotionProfileArc"=10, "Disabled"=15] ("Control Mode")
          # "Wait X miliseconds"
          # "Stop All Action"
          n67 = Wait (ms)(milliseconds to wait=u32 6000) -> ()  [unwired: 1 out]
          n68 = call <vilib>:"CTRE_Phoenix_MotorControl_Set.vi"("error in (no error)"=w207, "Output"=0.0, "Control Mode"=w205, "PhoenixMotorControlDevRef"=w208) -> ()  [unwired: 6 in, 2 out]
          n69 = call <vilib>:"WPI_MotorControlSetOutput.vi"("error in (no error)"=w210, "Output"=0.0, "MotorControlDevRef"=w211) -> ()  [unwired: 6 in, 3 out]
        }
        frame #4 {
          # "Stop Shooting and indexing\nGo for Mobility"
          n70 = while {
            shift-right: [w226] -> w213
            shift-left: w216 -> [w228]
            shift-right: [w225] -> w212
            shift-left: w215 -> [w227]
            tunnel: w214 -> [w217]
            stop <- w224 stop-if-true
            w223 = -0.4 ("Left axis value")
            # "Invert axis to flip back wheels\nnegative"
            n71 = call-poly <vilib>:"CTRE_Phoenix_MotorController_Get_TalonFX.vi"("PhoenixMotorControlDevRef"=w227, "error in"=w217) -> ("PhoenixMotorControlDevRef"=w225:T6, "Position (Raw Sensor Units)"=w219:i32)  [unwired: 10 in, 2 out]
            n72 = call <vilib>:"WPI_RobotDriveTankDrive.vi"("Right axis value"=w223, "Left axis value"=w223, "RobotDriveDevRef"=w228) -> ("RobotDriveDevRef"=w226:T5)  [unwired: 6 in, 2 out]
            n73 = Divide(x=w219, y=2048) -> (x/y=w220:dbl)
            n74 = Round To Nearest(number=w220) -> (nearest integer value=w218:dbl)
            n75 = Less Or Equal?(x=w218, y=-60) -> (x <= y?=w224:bool)
            n76 = local write "Talon FX LEFT Moter Encoders"(w218) -> ()
          }
        }
        frame #5 {
          w232 = 0.0 ("Left axis value")
          # "Stop all action"
          n77 = call <vilib>:"WPI_RobotDriveTankDrive.vi"("Right axis value"=w232, "Left axis value"=w232, "RobotDriveDevRef"=w231) -> ()  [unwired: 6 in, 3 out]
          n78 = call <vilib>:"CTRE_Phoenix_MotorControl_SetSelectedSensorPosition.vi"("New Sensor Position"=0, "PhoenixMotorControlDevRef"=w230) -> ()  [unwired: 8 in, 2 out]
        }
      }
    }
    frame "Left Position 3 Shoot 1 Mobility" {
      n79 = call <vilib>:"WPI_MotorControlRefNum Registry Get.vi"("refnum name"="Shooter Motors") -> ("error out"=w254:errorcluster, "MotorControlDevRef"=w255:T6)  [unwired: 9 in]
      n80 = call <vilib>:"CTRE_Phoenix_MotorControl_RefNumRegistryGet.vi"("refnum name"="Indexer") -> ("error out"=w256:errorcluster, "PhoenixMotorControlDevRef"=w257:T6)  [unwired: 9 in]
      n81 = call <vilib>:"WPI_RobotDriveRefNum Registry Get.vi"("refnum name"="Left and Right Motors") -> ("RobotDriveDevRef"=w249:T5)  [unwired: 9 in, 1 out]
      n82 = call <vilib>:"CTRE_Phoenix_MotorControl_RefNumRegistryGet.vi"("refnum name"="Left Motors") -> ("error out"=w250:errorcluster, "PhoenixMotorControlDevRef"=w251:T6)  [unwired: 9 in]
      n83 = call <vilib>:"CTRE_PigeonIMU_RefNumRegistryGet.vi"("refnum name"="Robot Angle") -> ("PigeonIMUDevRef"=w246:T12)  [unwired: 9 in, 1 out]
      n84 = flat-sequence {
        tunnel: [w291] -> w276
        tunnel: [w290] -> w275
        tunnel: [w289] -> w274
        tunnel: [w288] -> w273
        tunnel: [w280] -> w272
        tunnel: [w283] -> w271
        tunnel: [w282] -> w270
        tunnel: [w279] -> w269
        tunnel: w255 -> [w295]
        tunnel: w254 -> [w294]
        tunnel: w257 -> [w287]
        tunnel: w256 -> [w286]
        tunnel: w251 -> [w278]
        tunnel: w250 -> [w281]
        tunnel: w249 -> [w283]
        tunnel: w246 -> [w282]
        tunnel: w276 -> [w310]
        tunnel: w275 -> [w309]
        tunnel: [w308] -> w244
        tunnel: [w307] -> w243
        tunnel: [w305] -> w242
        tunnel: [w304] -> w241
        tunnel: w274 -> [w303]
        tunnel: w273 -> [w302]
        tunnel: [w299] -> w240
        tunnel: w272 -> [w298]
        tunnel: [w298] -> w238
        tunnel: [w297] -> w236
        tunnel: w271 -> [w297]
        tunnel: w270 -> [w296]
        tunnel: [w296] -> w234
        tunnel: w269 -> [w299]
        tunnel: w244 -> [w323]
        tunnel: w243 -> [w322]
        tunnel: w242 -> [w321]
        tunnel: w241 -> [w320]
        tunnel: w240 -> [w319]
        tunnel: [w319] -> w239
        tunnel: w238 -> [w318]
        tunnel: [w318] -> w237
        tunnel: w236 -> [w317]
        tunnel: [w317] -> w235
        tunnel: w234 -> [w316]
        tunnel: [w316] -> w233
        tunnel: w239 -> [w328]
        tunnel: w237 -> [w327]
        tunnel: w235 -> [w325]
        tunnel: w233 -> [w326]
        tunnel: [w326] -> w268
        tunnel: [w325] -> w267
        tunnel: [w324] -> w266
        tunnel: w268 -> [w343]
        tunnel: [w342] -> w265
        tunnel: w267 -> [w345]
        tunnel: [w345] -> w264
        tunnel: w266 -> [w344]
        tunnel: [w344] -> w263
        tunnel: w265 -> [w350]
        tunnel: w264 -> [w349]
        tunnel: [w347] -> w262
        tunnel: w263 -> [w346]
        tunnel: [w346] -> w261
        tunnel: w262 -> [w372]
        tunnel: [w372] -> w260
        tunnel: [w371] -> w259
        tunnel: w261 -> [w369]
        tunnel: w260 -> [w377]
        tunnel: w259 -> [w376]
        tunnel: [w375] -> w258
        tunnel: w258 -> [w396]
        frame #0 {
          w284 = T11 0 items=["PercentOutput"=0, "Position"=1, "Velocity"=2, "Current"=3, "Follower"=5, "MotionProfile"=6, "MotionMagic"=7, "MotionProfileArc"=10, "Disabled"=15] ("Control Mode")
          # "Rev up Shooter"
          n85 = call <vilib>:"CTRE_Phoenix_MotorControl_SetSelectedSensorPosition.vi"("error in (no error)"=w281, "New Sensor Position"=0, "PhoenixMotorControlDevRef"=w278) -> ("error out"=w280:errorcluster, "PhoenixMotorControlDevRef"=w279:T6)  [unwired: 7 in]
          n86 = call <vilib>:"WPI_MotorControlSetOutput.vi"("error in (no error)"=w294, "Output"=0.4, "MotorControlDevRef"=w295) -> ("error out"=w290:errorcluster, "MotorControlDevRef"=w291:T6)  [unwired: 6 in, 1 out]
          n87 = Wait (ms)(milliseconds to wait=u32 750) -> ()  [unwired: 1 out]
          n88 = call <vilib>:"CTRE_Phoenix_MotorControl_Set.vi"("error in (no error)"=w286, "Output"=0.0, "Control Mode"=w284, "PhoenixMotorControlDevRef"=w287) -> ("error out"=w288:errorcluster, "PhoenixMotorControlDevRef"=w289:T6)  [unwired: 6 in]
        }
        frame #1 {
          w300 = T11 0 items=["PercentOutput"=0, "Position"=1, "Velocity"=2, "Current"=3, "Follower"=5, "MotionProfile"=6, "MotionMagic"=7, "MotionProfileArc"=10, "Disabled"=15] ("Control Mode")
          # "Index and then Shoot"
          n89 = call <vilib>:"CTRE_Phoenix_MotorControl_Set.vi"("error in (no error)"=w302, "Output"=0.5, "Control Mode"=w300, "PhoenixMotorControlDevRef"=w303) -> ("error out"=w304:errorcluster, "PhoenixMotorControlDevRef"=w305:T6)  [unwired: 6 in]
          n90 = Wait (ms)(milliseconds to wait=u32 1500) -> ()  [unwired: 1 out]
          n91 = call <vilib>:"WPI_MotorControlSetOutput.vi"("error in (no error)"=w309, "Output"=0.4, "MotorControlDevRef"=w310) -> ("error out"=w307:errorcluster, "MotorControlDevRef"=w308:T6)  [unwired: 6 in, 1 out]
        }
        frame #2 {
          w314 = T11 0 items=["PercentOutput"=0, "Position"=1, "Velocity"=2, "Current"=3, "Follower"=5, "MotionProfile"=6, "MotionMagic"=7, "MotionProfileArc"=10, "Disabled"=15] ("Control Mode")
          # "Wait X miliseconds"
          n92 = Wait (ms)(milliseconds to wait=u32 5000) -> ()  [unwired: 1 out]
          n93 = call <vilib>:"WPI_MotorControlSetOutput.vi"("error in (no error)"=w322, "Output"=0.0, "MotorControlDevRef"=w323) -> ()  [unwired: 6 in, 3 out]
          n94 = call <vilib>:"CTRE_Phoenix_MotorControl_Set.vi"("error in (no error)"=w320, "Output"=0.0, "Control Mode"=w314, "PhoenixMotorControlDevRef"=w321) -> ()  [unwired: 6 in, 2 out]
        }
        frame #3 {
          # "Stop All Action Drive Back x distance"
          n95 = while {
            shift-right: [w338] -> _
            shift-left: w325 -> [w340]
            shift-right: [w337] -> w324
            shift-left: w328 -> [w339]
            tunnel: w327 -> [w329]
            stop <- w336 stop-if-true
            w335 = -0.4 ("Left axis value")
            # "Drive Back X Distance"
            n96 = call-poly <vilib>:"CTRE_Phoenix_MotorController_Get_TalonFX.vi"("PhoenixMotorControlDevRef"=w339, "error in"=w329) -> ("PhoenixMotorControlDevRef"=w337:T6, "Position (Raw Sensor Units)"=w331:i32)  [unwired: 10 in, 2 out]
            n97 = call <vilib>:"WPI_RobotDriveTankDrive.vi"("Right axis value"=w335, "Left axis value"=w335, "RobotDriveDevRef"=w340) -> ("RobotDriveDevRef"=w338:T5)  [unwired: 6 in, 2 out]
            n98 = Divide(x=w331, y=2048) -> (x/y=w332:dbl)
            n99 = Round To Nearest(number=w332) -> (nearest integer value=w330:dbl)
            n100 = Less Or Equal?(x=w330, y=-12) -> (x <= y?=w336:bool)
            n101 = local write "Talon FX LEFT Moter Encoders"(w330) -> ()
          }
        }
        frame #4 {
          n102 = call <vilib>:"CTRE_PigeonIMU_SetAccumZAngle.vi"("Angle (Deg)"=0.0, "PigeonIMUDevRef"=w343) -> ("PigeonIMUDevRef"=w342:T12)  [unwired: 8 in, 1 out]
        }
        frame #5 {
          # "Turn X Degrees"
          n103 = flat-sequence {
            tunnel: w350 -> [w353]
            tunnel: w349 -> [w352]
            tunnel: [w351] -> w348
            tunnel: w348 -> [w368]
            tunnel: [w366] -> w347
            frame #0 {
              # "Turn -90 degrees"
              n104 = while {
                shift-right: [w364] -> w351
                shift-left: w352 -> [w365]
                shift-right: [w357] -> _
                shift-left: w353 -> [w363]
                stop <- w360 stop-if-true
                n105 = call-poly <vilib>:"CTRE_Phoenix_Pigeon2_GetStatus.vi"("PigeonIMUDevRef"=w363) -> ("AccumGyro"=w362:cluster{"X":dbl, "Y":dbl, "Z":dbl}, "PigeonIMUDevRef"=w357:T12)  [unwired: 8 in, 1 out]
                n106 = call-poly <vilib>:"WPI_RobotDriveArcadeDrive.vi"("Y axis value"=0.0, "X axis value"=0.4, "RobotDriveDevRef"=w365) -> ("RobotDriveDevRef"=w364:T5)  [unwired: 6 in, 2 out]
                n107 = Unbundle(w362) -> ("X"=→"X":dbl, "Y"=→"Y":dbl, "Z"=w354:dbl)
                "Z" <- w354
                n108 = Less Or Equal?(x=w354, y=-40.0) -> (x <= y?=w360:bool)
              }
            }
            frame #1 {
              w367 = 0.0 ("Y axis value")
              # "Stop Turning"
              n109 = call-poly <vilib>:"WPI_RobotDriveArcadeDrive.vi"("Y axis value"=w367, "X axis value"=w367, "RobotDriveDevRef"=w368) -> ("RobotDriveDevRef"=w366:T5)  [unwired: 6 in, 2 out]
            }
          }
        }
        frame #6 {
          # "Reset Talon FX\nEncoder"
          n110 = call <vilib>:"CTRE_Phoenix_MotorControl_SetSelectedSensorPosition.vi"("New Sensor Position"=0, "PhoenixMotorControlDevRef"=w369) -> ("PhoenixMotorControlDevRef"=w371:T6)  [unwired: 8 in, 1 out]
        }
        frame #7 {
          n111 = flat-sequence {
            tunnel: w377 -> [w381]
            tunnel: w376 -> [w379]
            tunnel: [w380] -> w374
            tunnel: [w378] -> w373
            tunnel: [w395] -> w375
            tunnel: w374 -> [w393]
            tunnel: w373 -> [w395]
            frame #0 {
              # "Continue Mobility"
              n112 = while {
                shift-right: [w390] -> w380
                shift-left: w381 -> [w392]
                shift-right: [w389] -> w378
                shift-left: w379 -> [w391]
                stop <- w388 stop-if-true
                w387 = -0.4 ("Left axis value")
                # "Drive back X Revolution"
                n113 = call-poly <vilib>:"CTRE_Phoenix_MotorController_Get_TalonFX.vi"("PhoenixMotorControlDevRef"=w391) -> ("PhoenixMotorControlDevRef"=w389:T6, "Position (Raw Sensor Units)"=w383:i32)  [unwired: 11 in, 2 out]
                n114 = call <vilib>:"WPI_RobotDriveTankDrive.vi"("Right axis value"=w387, "Left axis value"=w387, "RobotDriveDevRef"=w392) -> ("RobotDriveDevRef"=w390:T5)  [unwired: 6 in, 2 out]
                n115 = Divide(x=w383, y=2048) -> (x/y=w384:dbl)
                n116 = Round To Nearest(number=w384) -> (nearest integer value=w382:dbl)
                n117 = Less Or Equal?(x=w382, y=-60) -> (x <= y?=w388:bool)
                n118 = local write "Talon FX LEFT Moter Encoders"(w382) -> ()
              }
            }
            frame #1 {
              w394 = 0.0 ("Left axis value")
              n119 = call <vilib>:"WPI_RobotDriveTankDrive.vi"("Right axis value"=w394, "Left axis value"=w394, "RobotDriveDevRef"=w393) -> ()  [unwired: 6 in, 3 out]
            }
          }
        }
        frame #8 {
          # "Stop Moving"
          n120 = call <vilib>:"CTRE_Phoenix_MotorControl_SetSelectedSensorPosition.vi"("New Sensor Position"=0, "PhoenixMotorControlDevRef"=w396) -> ()  [unwired: 8 in, 2 out]
        }
      }
    }
    frame "Right Postion 1 Shoot 1 Mobility" {
      n121 = call <vilib>:"WPI_MotorControlRefNum Registry Get.vi"("refnum name"="Shooter Motors") -> ("error out"=w421:errorcluster, "MotorControlDevRef"=w422:T6)  [unwired: 9 in]
      n122 = call <vilib>:"CTRE_Phoenix_MotorControl_RefNumRegistryGet.vi"("refnum name"="Indexer") -> ("error out"=w423:errorcluster, "PhoenixMotorControlDevRef"=w424:T6)  [unwired: 9 in]
      n123 = call <vilib>:"WPI_RobotDriveRefNum Registry Get.vi"("refnum name"="Left and Right Motors") -> ("RobotDriveDevRef"=w416:T5)  [unwired: 9 in, 1 out]
      n124 = call <vilib>:"CTRE_Phoenix_MotorControl_RefNumRegistryGet.vi"("refnum name"="Left Motors") -> ("error out"=w417:errorcluster, "PhoenixMotorControlDevRef"=w418:T6)  [unwired: 9 in]
      n125 = call <vilib>:"CTRE_PigeonIMU_RefNumRegistryGet.vi"("refnum name"="Robot Angle") -> ("PigeonIMUDevRef"=w413:T12)  [unwired: 9 in, 1 out]
      n126 = flat-sequence {
        tunnel: [w456] -> w441
        tunnel: [w455] -> w440
        tunnel: [w454] -> w439
        tunnel: [w453] -> w438
        tunnel: [w445] -> w437
        tunnel: [w448] -> w436
        tunnel: [w447] -> w435
        tunnel: [w444] -> w434
        tunnel: w422 -> [w460]
        tunnel: w421 -> [w459]
        tunnel: w424 -> [w452]
        tunnel: w423 -> [w451]
        tunnel: w418 -> [w443]
        tunnel: w417 -> [w446]
        tunnel: w416 -> [w448]
        tunnel: w413 -> [w447]
        tunnel: w441 -> [w475]
        tunnel: w440 -> [w474]
        tunnel: [w473] -> w409
        tunnel: [w472] -> w408
        tunnel: [w470] -> w407
        tunnel: [w469] -> w406
        tunnel: w439 -> [w468]
        tunnel: w438 -> [w467]
        tunnel: [w464] -> w405
        tunnel: w437 -> [w463]
        tunnel: [w463] -> w403
        tunnel: [w462] -> w401
        tunnel: w436 -> [w462]
        tunnel: w435 -> [w461]
        tunnel: [w461] -> w399
        tunnel: w434 -> [w464]
        tunnel: w409 -> [w488]
        tunnel: w408 -> [w487]
        tunnel: w407 -> [w486]
        tunnel: w406 -> [w485]
        tunnel: w405 -> [w484]
        tunnel: [w484] -> w404
        tunnel: w403 -> [w483]
        tunnel: [w483] -> w402
        tunnel: w401 -> [w482]
        tunnel: [w482] -> w400
        tunnel: w399 -> [w481]
        tunnel: [w481] -> w398
        tunnel: w404 -> [w492]
        tunnel: w402 -> [w491]
        tunnel: w400 -> [w489]
        tunnel: w398 -> [w493]
        tunnel: [w493] -> w433
        tunnel: [w490] -> w432
        tunnel: [w489] -> w411
        tunnel: w433 -> [w509]
        tunnel: [w508] -> w431
        tunnel: w432 -> [w510]
        tunnel: [w510] -> w430
        tunnel: w411 -> [w506]
        tunnel: [w506] -> w410
        tunnel: w431 -> [w515]
        tunnel: [w513] -> w429
        tunnel: w430 -> [w512]
        tunnel: [w512] -> w428
        tunnel: w410 -> [w511]
        tunnel: w429 -> [w537]
        tunnel: [w537] -> w427
        tunnel: [w536] -> w426
        tunnel: w428 -> [w534]
        tunnel: w427 -> [w542]
        tunnel: w426 -> [w541]
        tunnel: [w540] -> w425
        tunnel: w425 -> [w561]
        frame #0 {
          w449 = T11 0 items=["PercentOutput"=0, "Position"=1, "Velocity"=2, "Current"=3, "Follower"=5, "MotionProfile"=6, "MotionMagic"=7, "MotionProfileArc"=10, "Disabled"=15] ("Control Mode")
          # "Rev up Shooter"
          n127 = call <vilib>:"CTRE_Phoenix_MotorControl_SetSelectedSensorPosition.vi"("error in (no error)"=w446, "New Sensor Position"=0, "PhoenixMotorControlDevRef"=w443) -> ("error out"=w445:errorcluster, "PhoenixMotorControlDevRef"=w444:T6)  [unwired: 7 in]
          n128 = call <vilib>:"WPI_MotorControlSetOutput.vi"("error in (no error)"=w459, "Output"=0.4, "MotorControlDevRef"=w460) -> ("error out"=w455:errorcluster, "MotorControlDevRef"=w456:T6)  [unwired: 6 in, 1 out]
          n129 = Wait (ms)(milliseconds to wait=u32 750) -> ()  [unwired: 1 out]
          n130 = call <vilib>:"CTRE_Phoenix_MotorControl_Set.vi"("error in (no error)"=w451, "Output"=0.0, "Control Mode"=w449, "PhoenixMotorControlDevRef"=w452) -> ("error out"=w453:errorcluster, "PhoenixMotorControlDevRef"=w454:T6)  [unwired: 6 in]
        }
        frame #1 {
          w465 = T11 0 items=["PercentOutput"=0, "Position"=1, "Velocity"=2, "Current"=3, "Follower"=5, "MotionProfile"=6, "MotionMagic"=7, "MotionProfileArc"=10, "Disabled"=15] ("Control Mode")
          # "Index and then Shoot"
          n131 = call <vilib>:"CTRE_Phoenix_MotorControl_Set.vi"("error in (no error)"=w467, "Output"=0.5, "Control Mode"=w465, "PhoenixMotorControlDevRef"=w468) -> ("error out"=w469:errorcluster, "PhoenixMotorControlDevRef"=w470:T6)  [unwired: 6 in]
          n132 = Wait (ms)(milliseconds to wait=u32 1500) -> ()  [unwired: 1 out]
          n133 = call <vilib>:"WPI_MotorControlSetOutput.vi"("error in (no error)"=w474, "Output"=0.4, "MotorControlDevRef"=w475) -> ("error out"=w472:errorcluster, "MotorControlDevRef"=w473:T6)  [unwired: 6 in, 1 out]
        }
        frame #2 {
          w479 = T11 0 items=["PercentOutput"=0, "Position"=1, "Velocity"=2, "Current"=3, "Follower"=5, "MotionProfile"=6, "MotionMagic"=7, "MotionProfileArc"=10, "Disabled"=15] ("Control Mode")
          # "Wait X miliseconds"
          # "Stop All Action Drive Back x distance"
          n134 = Wait (ms)(milliseconds to wait=u32 0) -> ()  [unwired: 1 out]
          n135 = call <vilib>:"WPI_MotorControlSetOutput.vi"("error in (no error)"=w487, "Output"=0.0, "MotorControlDevRef"=w488) -> ()  [unwired: 6 in, 3 out]
          n136 = call <vilib>:"CTRE_Phoenix_MotorControl_Set.vi"("error in (no error)"=w485, "Output"=0.0, "Control Mode"=w479, "PhoenixMotorControlDevRef"=w486) -> ()  [unwired: 6 in, 2 out]
        }
        frame #3 {
          n137 = while {
            shift-right: [w503] -> _
            shift-left: w489 -> [w505]
            shift-right: [w502] -> w490
            shift-left: w492 -> [w504]
            tunnel: w491 -> [w494]
            stop <- w501 stop-if-true
            w500 = -0.4 ("Left axis value")
            # "Drive Back X Distance"
            n138 = call-poly <vilib>:"CTRE_Phoenix_MotorController_Get_TalonFX.vi"("PhoenixMotorControlDevRef"=w504, "error in"=w494) -> ("PhoenixMotorControlDevRef"=w502:T6, "Position (Raw Sensor Units)"=w496:i32)  [unwired: 10 in, 2 out]
            n139 = call <vilib>:"WPI_RobotDriveTankDrive.vi"("Right axis value"=w500, "Left axis value"=w500, "RobotDriveDevRef"=w505) -> ("RobotDriveDevRef"=w503:T5)  [unwired: 6 in, 2 out]
            n140 = Divide(x=w496, y=2048) -> (x/y=w497:dbl)
            n141 = Round To Nearest(number=w497) -> (nearest integer value=w495:dbl)
            n142 = Less Or Equal?(x=w495, y=-12) -> (x <= y?=w501:bool)
            n143 = local write "Talon FX LEFT Moter Encoders"(w495) -> ()
          }
        }
        frame #4 {
          n144 = call <vilib>:"CTRE_PigeonIMU_SetAccumZAngle.vi"("Angle (Deg)"=0.0, "PigeonIMUDevRef"=w509) -> ("PigeonIMUDevRef"=w508:T12)  [unwired: 8 in, 1 out]
        }
        frame #5 {
          # "Turn X Degrees"
          n145 = flat-sequence {
            tunnel: w515 -> [w518]
            tunnel: [w517] -> w514
            tunnel: w511 -> [w516]
            tunnel: w514 -> [w533]
            tunnel: [w531] -> w513
            frame #0 {
              # "Turn 40 degrees"
              n146 = while {
                shift-right: [w529] -> w517
                shift-left: w516 -> [w530]
                shift-right: [w522] -> _
                shift-left: w518 -> [w528]
                stop <- w525 stop-if-true
                # "Robot Angle"
                n147 = call-poly <vilib>:"CTRE_Phoenix_Pigeon2_GetStatus.vi"("PigeonIMUDevRef"=w528) -> ("AccumGyro"=w527:cluster{"X":dbl, "Y":dbl, "Z":dbl}, "PigeonIMUDevRef"=w522:T12)  [unwired: 8 in, 1 out]
                n148 = call-poly <vilib>:"WPI_RobotDriveArcadeDrive.vi"("Y axis value"=0.0, "X axis value"=-0.4, "RobotDriveDevRef"=w530) -> ("RobotDriveDevRef"=w529:T5)  [unwired: 6 in, 2 out]
                n149 = Unbundle(w527) -> ("X"=w519:dbl, "Y"=w520:dbl, "Z"=w521:dbl)
                n150 = Greater Or Equal?(x=w521, y=40.0) -> (x >= y?=w525:bool)
                n151 = local write "X"(w519) -> ()
                n152 = local write "Z"(w521) -> ()
                n153 = local write "Y"(w520) -> ()
              }
            }
            frame #1 {
              w532 = 0.0 ("Y axis value")
              # "Stop Turning"
              n154 = call-poly <vilib>:"WPI_RobotDriveArcadeDrive.vi"("Y axis value"=w532, "X axis value"=w532, "RobotDriveDevRef"=w533) -> ("RobotDriveDevRef"=w531:T5)  [unwired: 6 in, 2 out]
            }
          }
        }
        frame #6 {
          # "Reset Talon FX\nEncoder"
          n155 = call <vilib>:"CTRE_Phoenix_MotorControl_SetSelectedSensorPosition.vi"("New Sensor Position"=0, "PhoenixMotorControlDevRef"=w534) -> ("PhoenixMotorControlDevRef"=w536:T6)  [unwired: 8 in, 1 out]
        }
        frame #7 {
          n156 = flat-sequence {
            tunnel: w542 -> [w546]
            tunnel: w541 -> [w544]
            tunnel: [w545] -> w539
            tunnel: [w543] -> w538
            tunnel: [w560] -> w540
            tunnel: w539 -> [w558]
            tunnel: w538 -> [w560]
            frame #0 {
              # "Continue Mobility"
              n157 = while {
                shift-right: [w555] -> w545
                shift-left: w546 -> [w557]
                shift-right: [w554] -> w543
                shift-left: w544 -> [w556]
                stop <- w553 stop-if-true
                w552 = -0.4 ("Left axis value")
                # "Drive back X Revolution"
                n158 = call-poly <vilib>:"CTRE_Phoenix_MotorController_Get_TalonFX.vi"("PhoenixMotorControlDevRef"=w556) -> ("PhoenixMotorControlDevRef"=w554:T6, "Position (Raw Sensor Units)"=w548:i32)  [unwired: 11 in, 2 out]
                n159 = call <vilib>:"WPI_RobotDriveTankDrive.vi"("Right axis value"=w552, "Left axis value"=w552, "RobotDriveDevRef"=w557) -> ("RobotDriveDevRef"=w555:T5)  [unwired: 6 in, 2 out]
                n160 = Divide(x=w548, y=2048) -> (x/y=w549:dbl)
                n161 = Round To Nearest(number=w549) -> (nearest integer value=w547:dbl)
                n162 = Less Or Equal?(x=w547, y=-60) -> (x <= y?=w553:bool)
                n163 = local write "Talon FX LEFT Moter Encoders"(w547) -> ()
              }
            }
            frame #1 {
              w559 = 0.0 ("Left axis value")
              n164 = call <vilib>:"WPI_RobotDriveTankDrive.vi"("Right axis value"=w559, "Left axis value"=w559, "RobotDriveDevRef"=w558) -> ()  [unwired: 6 in, 3 out]
            }
          }
        }
        frame #8 {
          # "Stop Moving"
          n165 = call <vilib>:"CTRE_Phoenix_MotorControl_SetSelectedSensorPosition.vi"("New Sensor Position"=0, "PhoenixMotorControlDevRef"=w561) -> ()  [unwired: 8 in, 2 out]
        }
      }
    }
    frame "Center Position 2 Shoot 2" {
      # "Intake until limit switch is pressed"
      n166 = call <vilib>:"WPI_MotorControlRefNum Registry Get.vi"("refnum name"="Shooter Motors") -> ("error out"=w572:errorcluster, "MotorControlDevRef"=w573:T6)  [unwired: 9 in]
      n167 = call <vilib>:"WPI_RobotDriveRefNum Registry Get.vi"("refnum name"="Left and Right Motors") -> ("RobotDriveDevRef"=w571:T5)  [unwired: 9 in, 1 out]
      n168 = call <vilib>:"CTRE_Phoenix_MotorControl_RefNumRegistryGet.vi"("refnum name"="Left Motors") -> ("error out"=w569:errorcluster, "PhoenixMotorControlDevRef"=w570:T6)  [unwired: 9 in]
      n169 = call <vilib>:"CTRE_Phoenix_MotorControl_RefNumRegistryGet.vi"("refnum name"="intake") -> ("error out"=w567:errorcluster, "PhoenixMotorControlDevRef"=w568:T6)  [unwired: 9 in]
      n170 = call <vilib>:"WPI_SwitchRefNum Registry Get.vi"("refnum name"="Intake Limit") -> ("error out"=w566:errorcluster, "SwitchDevRef"=w565:T14)  [unwired: 9 in]
      n171 = call <vilib>:"CTRE_Phoenix_MotorControl_RefNumRegistryGet.vi"("refnum name"="Indexer") -> ("error out"=w563:errorcluster, "PhoenixMotorControlDevRef"=w564:T6)  [unwired: 9 in]
      n172 = flat-sequence {
        tunnel: w573 -> [w651]
        tunnel: w572 -> [w650]
        tunnel: [w647] -> w629
        tunnel: [w646] -> w628
        tunnel: [w645] -> w627
        tunnel: [w644] -> w626
        tunnel: w570 -> [w637]
        tunnel: [w639] -> w625
        tunnel: w569 -> [w640]
        tunnel: w571 -> [w641]
        tunnel: [w641] -> w624
        tunnel: [w638] -> w623
        tunnel: w567 -> [w635]
        tunnel: [w635] -> w622
        tunnel: w568 -> [w634]
        tunnel: [w634] -> w621
        tunnel: w565 -> [w633]
        tunnel: [w633] -> w620
        tunnel: w566 -> [w632]
        tunnel: [w632] -> w619
        tunnel: w564 -> [w631]
        tunnel: w563 -> [w630]
        tunnel: w629 -> [w669]
        tunnel: w628 -> [w668]
        tunnel: [w667] -> w618
        tunnel: [w666] -> w617
        tunnel: w627 -> [w664]
        tunnel: w626 -> [w663]
        tunnel: [w660] -> w616
        tunnel: w625 -> [w659]
        tunnel: [w659] -> w615
        tunnel: [w658] -> w614
        tunnel: w624 -> [w658]
        tunnel: w623 -> [w660]
        tunnel: w622 -> [w657]
        tunnel: [w657] -> w613
        tunnel: w621 -> [w656]
        tunnel: [w656] -> w612
        tunnel: w620 -> [w655]
        tunnel: [w655] -> w611
        tunnel: w619 -> [w654]
        tunnel: [w654] -> w610
        tunnel: [w653] -> w609
        tunnel: [w652] -> w608
        tunnel: w618 -> [w693]
        tunnel: w617 -> [w692]
        tunnel: w616 -> [w690]
        tunnel: w615 -> [w689]
        tunnel: w614 -> [w688]
        tunnel: [w688] -> w607
        tunnel: [w687] -> w606
        tunnel: w613 -> [w682]
        tunnel: w612 -> [w681]
        tunnel: w611 -> [w686]
        tunnel: w610 -> [w685]
        tunnel: [w684] -> w605
        tunnel: [w683] -> w604
        tunnel: w609 -> [w680]
        tunnel: w608 -> [w679]
        tunnel: [w677] -> w603
        tunnel: [w676] -> w602
        tunnel: [w675] -> w601
        tunnel: [w674] -> w600
        tunnel: [w673] -> w599
        tunnel: w607 -> [w757]
        tunnel: [w757] -> w598
        tunnel: w606 -> [w746]
        tunnel: w605 -> [w754]
        tunnel: w604 -> [w753]
        tunnel: w603 -> [w750]
        tunnel: w602 -> [w749]
        tunnel: [w748] -> w597
        tunnel: w601 -> [w748]
        tunnel: [w745] -> w596
        tunnel: [w744] -> w595
        tunnel: w600 -> [w744]
        tunnel: [w743] -> w594
        tunnel: w599 -> [w743]
        tunnel: [w742] -> w593
        tunnel: [w741] -> w592
        tunnel: w598 -> [_]
        tunnel: w597 -> [w769]
        tunnel: [w768] -> w591
        tunnel: w596 -> [w770]
        tunnel: w595 -> [w765]
        tunnel: w594 -> [w766]
        tunnel: [w764] -> w589
        tunnel: [w763] -> w590
        tunnel: [w762] -> w588
        tunnel: [w761] -> w587
        tunnel: w593 -> [w761]
        tunnel: [w760] -> w586
        tunnel: w592 -> [w760]
        tunnel: w591 -> [w793]
        tunnel: w590 -> [w803]
        tunnel: w589 -> [w801]
        tunnel: w588 -> [w794]
        tunnel: w587 -> [w798]
        tunnel: w586 -> [w797]
        tunnel: [w796] -> w585
        tunnel: [w795] -> w584
        tunnel: [w794] -> w583
        tunnel: [w793] -> w582
        tunnel: [w791] -> w581
        tunnel: [w790] -> w580
        tunnel: w585 -> [w811]
        tunnel: w584 -> [w810]
        tunnel: w583 -> [w809]
        tunnel: w582 -> [w808]
        tunnel: w581 -> [w805]
        tunnel: w580 -> [w804]
        frame #0 {
          w642 = T11 0 items=["PercentOutput"=0, "Position"=1, "Velocity"=2, "Current"=3, "Follower"=5, "MotionProfile"=6, "MotionMagic"=7, "MotionProfileArc"=10, "Disabled"=15] ("Control Mode")
          # "Rev up Shooter"
          n173 = call <vilib>:"CTRE_Phoenix_MotorControl_SetSelectedSensorPosition.vi"("error in (no error)"=w640, "New Sensor Position"=0, "PhoenixMotorControlDevRef"=w637) -> ("error out"=w639:errorcluster, "PhoenixMotorControlDevRef"=w638:T6)  [unwired: 7 in]
          n174 = call <vilib>:"WPI_MotorControlSetOutput.vi"("error in (no error)"=w650, "Output"=0.4, "MotorControlDevRef"=w651) -> ("error out"=w646:errorcluster, "MotorControlDevRef"=w647:T6)  [unwired: 6 in, 1 out]
          n175 = Wait (ms)(milliseconds to wait=u32 750) -> ()  [unwired: 1 out]
          n176 = call <vilib>:"CTRE_Phoenix_MotorControl_Set.vi"("error in (no error)"=w630, "Output"=0.0, "Control Mode"=w642, "PhoenixMotorControlDevRef"=w631) -> ("error out"=w644:errorcluster, "PhoenixMotorControlDevRef"=w645:T6)  [unwired: 6 in]
        }
        frame #1 {
          w661 = T11 0 items=["PercentOutput"=0, "Position"=1, "Velocity"=2, "Current"=3, "Follower"=5, "MotionProfile"=6, "MotionMagic"=7, "MotionProfileArc"=10, "Disabled"=15] ("Control Mode")
          # "Index and then Shoot"
          n177 = Wait (ms)(milliseconds to wait=u32 1500) -> ()  [unwired: 1 out]
          n178 = call <vilib>:"WPI_MotorControlSetOutput.vi"("error in (no error)"=w668, "Output"=0.4, "MotorControlDevRef"=w669) -> ("error out"=w666:errorcluster, "MotorControlDevRef"=w667:T6)  [unwired: 6 in, 1 out]
          n179 = call <vilib>:"CTRE_Phoenix_MotorControl_Set.vi"("error in (no error)"=w663, "Output"=0.5, "Control Mode"=w661, "PhoenixMotorControlDevRef"=w664) -> ("error out"=w652:errorcluster, "PhoenixMotorControlDevRef"=w653:T6)  [unwired: 6 in]
        }
        frame #2 {
          # "Stop Shooter Drive Back x distance and Intake"
          n180 = while {
            shift-right: [w733] -> w684
            shift-left: w681 -> [w740]
            shift-right: [w732] -> w683
            shift-left: w682 -> [w739]
            tunnel: w686 -> [w729]
            tunnel: w685 -> [w728]
            tunnel: [w727] -> w678
            stop <- w727 stop-if-true
            w731 = 1.0 ("x")
            w734 = T11 0 items=["PercentOutput"=0, "Position"=1, "Velocity"=2, "Current"=3, "Follower"=5, "MotionProfile"=6, "MotionMagic"=7, "MotionProfileArc"=10, "Disabled"=15] ("Control Mode")
            n181 = call <vilib>:"WPI_SwitchGetLimitValue.vi"("error in (no error)"=w728, "SwitchDevRef"=w729) -> ("Switch Pressed"=w727:bool)  [unwired: 7 in, 2 out]
            "Limit Switch" <- w727
            n182 = In Range and Coerce(upper limit=0.0, x=w731, lower limit=-1.0) -> (coerced(x)=w738:dbl)  [unwired: 1 out]
            n183 = Select(t=w738, s=w727, f=w731) -> (s? t:f=w735:dbl)
            n184 = Wait (ms)(milliseconds to wait=u32 20) -> ()  [unwired: 1 out]
            n185 = call <vilib>:"CTRE_Phoenix_MotorControl_Set.vi"("error in (no error)"=w739, "Output"=w735, "Control Mode"=w734, "PhoenixMotorControlDevRef"=w740) -> ("error out"=w732:errorcluster, "PhoenixMotorControlDevRef"=w733:T6)  [unwired: 6 in]
          }
          n186 = while {
            shift-right: [w719] -> w677
            shift-left: w680 -> [w726]
            shift-right: [w718] -> w676
            shift-left: w679 -> [w725]
            tunnel: w678 -> [w715]
            stop <- w715 stop-if-true
            w717 = 0.5 ("x")
            w720 = T11 0 items=["PercentOutput"=0, "Position"=1, "Velocity"=2, "Current"=3, "Follower"=5, "MotionProfile"=6, "MotionMagic"=7, "MotionProfileArc"=10, "Disabled"=15] ("Control Mode")
            n187 = In Range and Coerce(upper limit=0.0, x=w717, lower limit=-1.0) -> (coerced(x)=w724:dbl)  [unwired: 1 out]
            n188 = Select(t=w724, s=w715, f=w717) -> (s? t:f=w721:dbl)
            n189 = Wait (ms)(milliseconds to wait=u32 20) -> ()  [unwired: 1 out]
            n190 = call <vilib>:"CTRE_Phoenix_MotorControl_Set.vi"("error in (no error)"=w725, "Output"=w721, "Control Mode"=w720, "PhoenixMotorControlDevRef"=w726) -> ("error out"=w718:errorcluster, "PhoenixMotorControlDevRef"=w719:T6)  [unwired: 6 in]
          }
          n191 = flat-sequence {
            tunnel: w690 -> [w698]
            tunnel: w689 -> [w697]
            tunnel: w688 -> [w696]
            tunnel: [w695] -> w672
            tunnel: [w694] -> w671
            tunnel: [w712] -> w675
            tunnel: [w714] -> w687
            tunnel: w672 -> [w714]
            tunnel: w671 -> [w711]
            frame #0 {
              n192 = while {
                shift-right: [w708] -> w694
                shift-left: w696 -> [w710]
                shift-right: [w707] -> w695
                shift-left: w698 -> [w709]
                tunnel: w697 -> [w699]
                stop <- w706 stop-if-true
                w705 = -0.5 ("Left axis value")
                # "Drive Back X Distance"
                n193 = call-poly <vilib>:"CTRE_Phoenix_MotorController_Get_TalonFX.vi"("PhoenixMotorControlDevRef"=w709, "error in"=w699) -> ("PhoenixMotorControlDevRef"=w707:T6, "Position (Raw Sensor Units)"=w701:i32)  [unwired: 10 in, 2 out]
                n194 = call <vilib>:"WPI_RobotDriveTankDrive.vi"("Right axis value"=w705, "Left axis value"=w705, "RobotDriveDevRef"=w710) -> ("RobotDriveDevRef"=w708:T5)  [unwired: 6 in, 2 out]
                n195 = Divide(x=w701, y=2048) -> (x/y=w702:dbl)
                n196 = Round To Nearest(number=w702) -> (nearest integer value=w700:dbl)
                n197 = Less Or Equal?(x=w700, y=-40) -> (x <= y?=w706:bool)
                n198 = local write "Talon FX LEFT Moter Encoders"(w700) -> ()
              }
            }
            frame #1 {
              w713 = 0.0 ("Left axis value")
              n199 = call <vilib>:"WPI_RobotDriveTankDrive.vi"("Right axis value"=w713, "Left axis value"=w713, "RobotDriveDevRef"=w711) -> ("RobotDriveDevRef"=w712:T5)  [unwired: 6 in, 2 out]
            }
          }
          n200 = call <vilib>:"WPI_MotorControlSetOutput.vi"("error in (no error)"=w692, "Output"=0.0, "MotorControlDevRef"=w693) -> ("error out"=w674:errorcluster, "MotorControlDevRef"=w673:T6)  [unwired: 6 in, 1 out]
        }
        frame #3 {
          w751 = T11 0 items=["PercentOutput"=0, "Position"=1, "Velocity"=2, "Current"=3, "Follower"=5, "MotionProfile"=6, "MotionMagic"=7, "MotionProfileArc"=10, "Disabled"=15] ("Control Mode")
          w755 = T11 0 items=["PercentOutput"=0, "Position"=1, "Velocity"=2, "Current"=3, "Follower"=5, "MotionProfile"=6, "MotionMagic"=7, "MotionProfileArc"=10, "Disabled"=15] ("Control Mode")
          # "Reset Drive Train Enoder"
          # "Stop Indexing"
          # "Stop Intaking"
          n201 = call <vilib>:"CTRE_Phoenix_MotorControl_SetSelectedSensorPosition.vi"("New Sensor Position"=0, "PhoenixMotorControlDevRef"=w746) -> ("PhoenixMotorControlDevRef"=w745:T6)  [unwired: 8 in, 1 out]
          n202 = call <vilib>:"CTRE_Phoenix_MotorControl_Set.vi"("error in (no error)"=w753, "Output"=0.0, "Control Mode"=w755, "PhoenixMotorControlDevRef"=w754) -> ()  [unwired: 6 in, 2 out]
          n203 = call <vilib>:"CTRE_Phoenix_MotorControl_Set.vi"("error in (no error)"=w749, "Output"=0.0, "Control Mode"=w751, "PhoenixMotorControlDevRef"=w750) -> ("error out"=w741:errorcluster, "PhoenixMotorControlDevRef"=w742:T6)  [unwired: 6 in]
        }
        frame #4 {
          # "Rev up shooter and Drive back x distance"
          n204 = flat-sequence {
            tunnel: w770 -> [w774]
            tunnel: w769 -> [w773]
            tunnel: [w772] -> w759
            tunnel: [w771] -> w758
            tunnel: [w789] -> w762
            tunnel: [w787] -> w768
            tunnel: w759 -> [w786]
            tunnel: w758 -> [w789]
            frame #0 {
              # "drive towards speaker"
              n205 = while {
                shift-right: [w783] -> w772
                shift-left: w773 -> [w785]
                shift-right: [w782] -> w771
                shift-left: w774 -> [w784]
                stop <- w781 stop-if-true
                w780 = 0.5 ("Left axis value")
                # "Drive Back X Distance"
                n206 = call-poly <vilib>:"CTRE_Phoenix_MotorController_Get_TalonFX.vi"("PhoenixMotorControlDevRef"=w784) -> ("PhoenixMotorControlDevRef"=w782:T6, "Position (Raw Sensor Units)"=w776:i32)  [unwired: 11 in, 2 out]
                n207 = call <vilib>:"WPI_RobotDriveTankDrive.vi"("Right axis value"=w780, "Left axis value"=w780, "RobotDriveDevRef"=w785) -> ("RobotDriveDevRef"=w783:T5)  [unwired: 6 in, 2 out]
                n208 = Divide(x=w776, y=2048) -> (x/y=w777:dbl)
                n209 = Round To Nearest(number=w777) -> (nearest integer value=w775:dbl)
                n210 = Greater Or Equal?(x=w775, y=38) -> (x >= y?=w781:bool)
                n211 = local write "Talon FX LEFT Moter Encoders"(w775) -> ()
              }
            }
            frame #1 {
              w788 = 0.0 ("Left axis value")
              n212 = call <vilib>:"WPI_RobotDriveTankDrive.vi"("Right axis value"=w788, "Left axis value"=w788, "RobotDriveDevRef"=w786) -> ("RobotDriveDevRef"=w787:T5)  [unwired: 6 in, 2 out]
            }
          }
          n213 = call <vilib>:"WPI_MotorControlSetOutput.vi"("error in (no error)"=w765, "Output"=0.4, "MotorControlDevRef"=w766) -> ("error out"=w763:errorcluster, "MotorControlDevRef"=w764:T6)  [unwired: 6 in, 1 out]
        }
        frame #5 {
          w799 = T11 0 items=["PercentOutput"=0, "Position"=1, "Velocity"=2, "Current"=3, "Follower"=5, "MotionProfile"=6, "MotionMagic"=7, "MotionProfileArc"=10, "Disabled"=15] ("Control Mode")
          # "Index to shoot"
          # "Shoot Note"
          n214 = call <vilib>:"CTRE_Phoenix_MotorControl_Set.vi"("error in (no error)"=w797, "Output"=0.5, "Control Mode"=w799, "PhoenixMotorControlDevRef"=w798) -> ("error out"=w790:errorcluster, "PhoenixMotorControlDevRef"=w791:T6)  [unwired: 6 in]
          n215 = call <vilib>:"WPI_MotorControlSetOutput.vi"("error in (no error)"=w803, "Output"=0.4, "MotorControlDevRef"=w801) -> ("error out"=w795:errorcluster, "MotorControlDevRef"=w796:T6)  [unwired: 6 in, 1 out]
          n216 = Wait (ms)(milliseconds to wait=u32 1500) -> ()  [unwired: 1 out]
        }
        frame #6 {
          w806 = T11 0 items=["PercentOutput"=0, "Position"=1, "Velocity"=2, "Current"=3, "Follower"=5, "MotionProfile"=6, "MotionMagic"=7, "MotionProfileArc"=10, "Disabled"=15] ("Control Mode")
          w814 = 0.0 ("Left axis value")
          # "Stop indexing"
          # "Stop All Action"
          # "Stop Moving"
          n217 = call <vilib>:"WPI_RobotDriveTankDrive.vi"("Right axis value"=w814, "Left axis value"=w814, "RobotDriveDevRef"=w808) -> ()  [unwired: 6 in, 3 out]
          n218 = call <vilib>:"CTRE_Phoenix_MotorControl_SetSelectedSensorPosition.vi"("New Sensor Position"=0, "PhoenixMotorControlDevRef"=w809) -> ()  [unwired: 8 in, 2 out]
          n219 = call <vilib>:"WPI_MotorControlSetOutput.vi"("error in (no error)"=w810, "Output"=0.0, "MotorControlDevRef"=w811) -> ()  [unwired: 6 in, 3 out]
          n220 = call <vilib>:"CTRE_Phoenix_MotorControl_Set.vi"("error in (no error)"=w804, "Output"=0.0, "Control Mode"=w806, "PhoenixMotorControlDevRef"=w805) -> ()  [unwired: 6 in, 2 out]
        }
      }
    }
    frame "Right Postion 1 Shoot 2" {
      n221 = call <vilib>:"WPI_MotorControlRefNum Registry Get.vi"("refnum name"="Shooter Motors") -> ("error out"=w819:errorcluster, "MotorControlDevRef"=w818:T6)  [unwired: 9 in]
      n222 = call <vilib>:"CTRE_PigeonIMU_RefNumRegistryGet.vi"("refnum name"="Robot Angle") -> ("error out"=w815:errorcluster, "PigeonIMUDevRef"=w816:T12)  [unwired: 9 in]
      n223 = call <vilib>:"WPI_RobotDriveRefNum Registry Get.vi"("refnum name"="Left and Right Motors") -> ("RobotDriveDevRef"=w820:T5)  [unwired: 9 in, 1 out]
      n224 = call <vilib>:"CTRE_Phoenix_MotorControl_RefNumRegistryGet.vi"("refnum name"="Left Motors") -> ("error out"=w822:errorcluster, "PhoenixMotorControlDevRef"=w821:T6)  [unwired: 9 in]
      n225 = call <vilib>:"CTRE_Phoenix_MotorControl_RefNumRegistryGet.vi"("refnum name"="intake") -> ("error out"=w824:errorcluster, "PhoenixMotorControlDevRef"=w823:T6)  [unwired: 9 in]
      n226 = call <vilib>:"WPI_SwitchRefNum Registry Get.vi"("refnum name"="Intake Limit") -> ("error out"=w827:errorcluster, "SwitchDevRef"=w828:T14)  [unwired: 9 in]
      n227 = call <vilib>:"CTRE_Phoenix_MotorControl_RefNumRegistryGet.vi"("refnum name"="Indexer") -> ("error out"=w825:errorcluster, "PhoenixMotorControlDevRef"=w826:T6)  [unwired: 9 in]
      n228 = flat-sequence {
        tunnel: w818 -> [w955]
        tunnel: w819 -> [w954]
        tunnel: [w951] -> w928
        tunnel: [w950] -> w927
        tunnel: [w949] -> w926
        tunnel: [w948] -> w925
        tunnel: w821 -> [w942]
        tunnel: [w944] -> w924
        tunnel: w822 -> [w945]
        tunnel: [w934] -> _
        tunnel: [w934] -> w923
        tunnel: [w943] -> w922
        tunnel: [w936] -> _
        tunnel: [w936] -> w921
        tunnel: [w935] -> _
        tunnel: [w935] -> w920
        tunnel: w828 -> [w940]
        tunnel: [w940] -> w919
        tunnel: w827 -> [w939]
        tunnel: [w939] -> w918
        tunnel: [w937] -> _
        tunnel: w825 -> [w938]
        tunnel: w826 -> [w937]
        tunnel: w824 -> [w936]
        tunnel: w823 -> [w935]
        tunnel: w820 -> [w934]
        tunnel: w816 -> [w933]
        tunnel: w815 -> [w932]
        tunnel: [w930] -> w917
        tunnel: [w929] -> w916
        tunnel: w928 -> [w975]
        tunnel: w927 -> [w974]
        tunnel: [w973] -> w915
        tunnel: [w972] -> w914
        tunnel: w926 -> [w970]
        tunnel: w925 -> [w969]
        tunnel: [w966] -> w913
        tunnel: w924 -> [w965]
        tunnel: [w965] -> w912
        tunnel: [w964] -> w911
        tunnel: w923 -> [w964]
        tunnel: w922 -> [w966]
        tunnel: w921 -> [w963]
        tunnel: [w963] -> w910
        tunnel: w920 -> [w962]
        tunnel: [w962] -> w909
        tunnel: w919 -> [w961]
        tunnel: [w961] -> w908
        tunnel: w918 -> [w960]
        tunnel: [w960] -> w907
        tunnel: [w959] -> w906
        tunnel: [w958] -> w905
        tunnel: w917 -> [w957]
        tunnel: w916 -> [w956]
        tunnel: [w957] -> w904
        tunnel: [w956] -> w903
        tunnel: w915 -> [w998]
        tunnel: w914 -> [w997]
        tunnel: w913 -> [w995]
        tunnel: w912 -> [w994]
        tunnel: w911 -> [w993]
        tunnel: w910 -> [w979]
        tunnel: w909 -> [w980]
        tunnel: w908 -> [w985]
        tunnel: w907 -> [w984]
        tunnel: w906 -> [w991]
        tunnel: w905 -> [w990]
        tunnel: [w992] -> w902
        tunnel: [w989] -> w901
        tunnel: w904 -> [w989]
        tunnel: [w988] -> w900
        tunnel: w903 -> [w988]
        tunnel: [w987] -> w899
        tunnel: [w986] -> w898
        tunnel: [w985] -> w897
        tunnel: [w984] -> w896
        tunnel: [w980] -> w895
        tunnel: [w979] -> w894
        tunnel: [w983] -> w893
        tunnel: [w982] -> w892
        tunnel: [w981] -> w891
        tunnel: w902 -> [w1026]
        tunnel: [w1016] -> w890
        tunnel: [w1025] -> w889
        tunnel: w901 -> [w1024]
        tunnel: w900 -> [w1023]
        tunnel: [w1022] -> w888
        tunnel: w899 -> [w1022]
        tunnel: [w1021] -> w887
        tunnel: w898 -> [w1021]
        tunnel: [w1020] -> w886
        tunnel: w897 -> [w1020]
        tunnel: w896 -> [w1019]
        tunnel: [w1019] -> w885
        tunnel: [w1018] -> w884
        tunnel: w895 -> [w1018]
        tunnel: w894 -> [w1017]
        tunnel: [w1017] -> w883
        tunnel: w893 -> [w1016]
        tunnel: w892 -> [_]
        tunnel: w891 -> [w1011]
        tunnel: [w1014] -> w882
        tunnel: [w1012] -> w881
        tunnel: [w1011] -> w880
        tunnel: w890 -> [w1057]
        tunnel: [w1056] -> w879
        tunnel: w889 -> [w1054]
        tunnel: [w1054] -> w878
        tunnel: w888 -> [w1063]
        tunnel: [w1063] -> w877
        tunnel: w887 -> [w1062]
        tunnel: [w1062] -> w876
        tunnel: w886 -> [w1061]
        tunnel: [w1061] -> w875
        tunnel: w885 -> [w1060]
        tunnel: [w1060] -> w874
        tunnel: w884 -> [w1059]
        tunnel: [w1059] -> w873
        tunnel: w883 -> [w1058]
        tunnel: [w1058] -> w872
        tunnel: w882 -> [w1053]
        tunnel: [w1053] -> w871
        tunnel: [w1052] -> w870
        tunnel: w881 -> [w1052]
        tunnel: [w1051] -> w869
        tunnel: w880 -> [w1051]
        tunnel: w879 -> [w1072]
        tunnel: w878 -> [w1071]
        tunnel: w877 -> [w1077]
        tunnel: w876 -> [w1078]
        tunnel: w875 -> [w1080]
        tunnel: w874 -> [w1079]
        tunnel: w873 -> [w1082]
        tunnel: w872 -> [w1081]
        tunnel: [w1076] -> w868
        tunnel: [w1075] -> w867
        tunnel: [w1073] -> w866
        tunnel: [w1074] -> w865
        tunnel: [w1069] -> w864
        tunnel: [w1067] -> w863
        tunnel: w871 -> [w1066]
        tunnel: [w1066] -> w862
        tunnel: w870 -> [w1065]
        tunnel: [w1065] -> w861
        tunnel: [w1064] -> w860
        tunnel: w869 -> [w1064]
        tunnel: w868 -> [w1137]
        tunnel: [w1137] -> w859
        tunnel: w867 -> [w1136]
        tunnel: [w1136] -> w858
        tunnel: w866 -> [w1135]
        tunnel: [w1135] -> w857
        tunnel: w865 -> [w1134]
        tunnel: [w1134] -> w856
        tunnel: w864 -> [w1133]
        tunnel: [w1133] -> w855
        tunnel: w863 -> [w1132]
        tunnel: [w1132] -> w854
        tunnel: w862 -> [w1129]
        tunnel: w861 -> [w1128]
        tunnel: w860 -> [w1131]
        tunnel: [w1131] -> w853
        tunnel: [w1127] -> w852
        tunnel: [w1126] -> w851
        tunnel: w859 -> [w1152]
        tunnel: w858 -> [w1151]
        tunnel: w857 -> [w1150]
        tunnel: w856 -> [w1149]
        tunnel: w855 -> [w1140]
        tunnel: w854 -> [w1139]
        tunnel: [w1146] -> w850
        tunnel: w853 -> [w1146]
        tunnel: [w1145] -> w849
        tunnel: [w1144] -> w848
        tunnel: w852 -> [w1142]
        tunnel: w851 -> [w1141]
        tunnel: [w1139] -> w847
        tunnel: [w1138] -> w846
        tunnel: w850 -> [w1178]
        tunnel: [w1178] -> w845
        tunnel: w849 -> [w1177]
        tunnel: [w1177] -> w844
        tunnel: w848 -> [w1176]
        tunnel: [w1176] -> w843
        tunnel: [w1174] -> w842
        tunnel: w847 -> [w1173]
        tunnel: w846 -> [w1172]
        tunnel: [w1172] -> w841
        tunnel: [w1179] -> w838
        tunnel: w845 -> [w1186]
        tunnel: [w1185] -> w839
        tunnel: w844 -> [w1185]
        tunnel: w843 -> [w1184]
        tunnel: [w1184] -> w840
        tunnel: w842 -> [w1182]
        tunnel: w841 -> [w1181]
        tunnel: [w1207] -> w835
        tunnel: [w1204] -> w836
        tunnel: w840 -> [w1205]
        tunnel: w839 -> [w1206]
        tunnel: w838 -> [w1211]
        tunnel: [w1210] -> w837
        tunnel: w837 -> [w1214]
        tunnel: w836 -> [w1217]
        tunnel: w835 -> [w1218]
        frame #0 {
          w946 = T11 0 items=["PercentOutput"=0, "Position"=1, "Velocity"=2, "Current"=3, "Follower"=5, "MotionProfile"=6, "MotionMagic"=7, "MotionProfileArc"=10, "Disabled"=15] ("Control Mode")
          # "Rev up Shooter"
          n229 = call <vilib>:"CTRE_PigeonIMU_SetAccumZAngle.vi"("error in (no error)"=w932, "Angle (Deg)"=0.0, "PigeonIMUDevRef"=w933) -> ("error out"=w929:errorcluster, "PigeonIMUDevRef"=w930:T12)  [unwired: 7 in]
          n230 = call <vilib>:"CTRE_Phoenix_MotorControl_SetSelectedSensorPosition.vi"("error in (no error)"=w945, "New Sensor Position"=0, "PhoenixMotorControlDevRef"=w942) -> ("error out"=w944:errorcluster, "PhoenixMotorControlDevRef"=w943:T6)  [unwired: 7 in]
          n231 = call <vilib>:"WPI_MotorControlSetOutput.vi"("error in (no error)"=w954, "Output"=0.4, "MotorControlDevRef"=w955) -> ("error out"=w950:errorcluster, "MotorControlDevRef"=w951:T6)  [unwired: 6 in, 1 out]
          n232 = Wait (ms)(milliseconds to wait=u32 750) -> ()  [unwired: 1 out]
          n233 = call <vilib>:"CTRE_Phoenix_MotorControl_Set.vi"("error in (no error)"=w938, "Output"=0.0, "Control Mode"=w946, "PhoenixMotorControlDevRef"=w937) -> ("error out"=w948:errorcluster, "PhoenixMotorControlDevRef"=w949:T6)  [unwired: 6 in]
        }
        frame #1 {
          w967 = T11 0 items=["PercentOutput"=0, "Position"=1, "Velocity"=2, "Current"=3, "Follower"=5, "MotionProfile"=6, "MotionMagic"=7, "MotionProfileArc"=10, "Disabled"=15] ("Control Mode")
          # "Index and then Shoot"
          n234 = Wait (ms)(milliseconds to wait=u32 1500) -> ()  [unwired: 1 out]
          n235 = call <vilib>:"WPI_MotorControlSetOutput.vi"("error in (no error)"=w974, "Output"=0.4, "MotorControlDevRef"=w975) -> ("error out"=w972:errorcluster, "MotorControlDevRef"=w973:T6)  [unwired: 6 in, 1 out]
          n236 = call <vilib>:"CTRE_Phoenix_MotorControl_Set.vi"("error in (no error)"=w969, "Output"=0.5, "Control Mode"=w967, "PhoenixMotorControlDevRef"=w970) -> ("error out"=w958:errorcluster, "PhoenixMotorControlDevRef"=w959:T6)  [unwired: 6 in]
        }
        frame #2 {
          w978 = T11 0 items=["PercentOutput"=0, "Position"=1, "Velocity"=2, "Current"=3, "Follower"=5, "MotionProfile"=6, "MotionMagic"=7, "MotionProfileArc"=10, "Disabled"=15] ("Control Mode")
          # "Stop Indexing/intaking"
          # "3)Stop index and shooter and drive back a little"
          n237 = call <vilib>:"CTRE_Phoenix_MotorControl_Set.vi"("error in (no error)"=w990, "Output"=0.0, "Control Mode"=w978, "PhoenixMotorControlDevRef"=w991) -> ("error out"=w987:errorcluster, "PhoenixMotorControlDevRef"=w986:T6)  [unwired: 6 in]
          n238 = while {
            shift-right: [w1008] -> w992
            shift-left: w993 -> [w1010]
            shift-right: [w1007] -> w983
            shift-left: w995 -> [w1009]
            tunnel: w994 -> [w1000]
            stop <- w1006 stop-if-true
            w1005 = -0.4 ("Left axis value")
            # "Drive Back X Distance"
            n239 = call-poly <vilib>:"CTRE_Phoenix_MotorController_Get_TalonFX.vi"("PhoenixMotorControlDevRef"=w1009, "error in"=w1000) -> ("PhoenixMotorControlDevRef"=w1007:T6, "Position (Raw Sensor Units)"=w1001:i32)  [unwired: 10 in, 2 out]
            n240 = call <vilib>:"WPI_RobotDriveTankDrive.vi"("Right axis value"=w1005, "Left axis value"=w1005, "RobotDriveDevRef"=w1010) -> ("RobotDriveDevRef"=w1008:T5)  [unwired: 6 in, 2 out]
            n241 = Divide(x=w1001, y=2048) -> (x/y=w1002:dbl)
            n242 = Round To Nearest(number=w1002) -> (nearest integer value=w999:dbl)
            n243 = Less Or Equal?(x=w999, y=-12) -> (x <= y?=w1006:bool)
            n244 = local write "Talon FX LEFT Moter Encoders"(w999) -> ()
          }
          n245 = call <vilib>:"WPI_MotorControlSetOutput.vi"("error in (no error)"=w997, "Output"=0.0, "MotorControlDevRef"=w998) -> ("error out"=w982:errorcluster, "MotorControlDevRef"=w981:T6)  [unwired: 6 in, 1 out]
        }
        frame #3 {
          # "Turn X Degrees"
          n246 = flat-sequence {
            tunnel: [w1033] -> w1027
            tunnel: w1026 -> [w1032]
            tunnel: w1024 -> [w1031]
            tunnel: w1023 -> [w1030]
            tunnel: [w1029] -> w1015
            tunnel: [w1028] -> w1013
            tunnel: w1027 -> [w1050]
            tunnel: [w1049] -> w1025
            tunnel: w1015 -> [w1046]
            tunnel: [w1047] -> w1014
            tunnel: w1013 -> [w1047]
            tunnel: [w1046] -> w1012
            frame #0 {
              # "Turn -45 degrees"
              n247 = while {
                shift-right: [w1044] -> w1033
                shift-left: w1032 -> [w1045]
                shift-right: [w1037] -> w1029
                shift-left: w1031 -> [w1043]
                tunnel: w1030 -> [w1036]
                tunnel: [w1035] -> w1028
                stop <- w1040 stop-if-true
                n248 = call-poly <vilib>:"CTRE_Phoenix_Pigeon2_GetStatus.vi"("error in (no error)"=w1036, "PigeonIMUDevRef"=w1043) -> ("error out"=w1035:errorcluster, "AccumGyro"=w1042:cluster{"X":dbl, "Y":dbl, "Z":dbl}, "PigeonIMUDevRef"=w1037:T12)  [unwired: 7 in]
                n249 = call-poly <vilib>:"WPI_RobotDriveArcadeDrive.vi"("Y axis value"=0.0, "X axis value"=-0.4, "RobotDriveDevRef"=w1045) -> ("RobotDriveDevRef"=w1044:T5)  [unwired: 6 in, 2 out]
                n250 = Unbundle(w1042) -> ("Z"=w1034:dbl)  [unwired: 2 out]
                n251 = Greater Or Equal?(x=w1034, y=23.0) -> (x >= y?=w1040:bool)
                n252 = local write "Z"(w1034) -> ()
              }
            }
            frame #1 {
              w1048 = 0.0 ("Y axis value")
              # "Stop Turning"
              n253 = call-poly <vilib>:"WPI_RobotDriveArcadeDrive.vi"("Y axis value"=w1048, "X axis value"=w1048, "RobotDriveDevRef"=w1050) -> ("RobotDriveDevRef"=w1049:T5)  [unwired: 6 in, 2 out]
            }
          }
        }
        frame #4 {
          n254 = call <vilib>:"CTRE_Phoenix_MotorControl_SetSelectedSensorPosition.vi"("New Sensor Position"=0, "PhoenixMotorControlDevRef"=w1057) -> ("PhoenixMotorControlDevRef"=w1056:T6)  [unwired: 8 in, 1 out]
        }
        frame #5 {
          # "5)Drive x distance and run indexer/intake"
          n255 = while {
            shift-right: [w1118] -> w1076
            shift-left: w1082 -> [w1124]
            shift-right: [w1117] -> w1075
            shift-left: w1081 -> [w1123]
            tunnel: w1080 -> [w1114]
            tunnel: w1079 -> [w1113]
            tunnel: w1078 -> [w1107]
            tunnel: w1077 -> [w1106]
            tunnel: [w1105] -> w1073
            tunnel: [w1104] -> w1074
            stop <- w1103 stop-if-true
            w1108 = 0.5 ("x")
            w1116 = 1.0 ("x")
            w1102 = T11 0 items=["PercentOutput"=0, "Position"=1, "Velocity"=2, "Current"=3, "Follower"=5, "MotionProfile"=6, "MotionMagic"=7, "MotionProfileArc"=10, "Disabled"=15] ("Control Mode")
            n256 = call <vilib>:"WPI_SwitchGetLimitValue.vi"("error in (no error)"=w1113, "SwitchDevRef"=w1114) -> ("Switch Pressed"=w1103:bool)  [unwired: 7 in, 2 out]
            n257 = local write "Limit Switch"(w1103) -> ()
            n258 = In Range and Coerce(upper limit=0.0, x=w1116, lower limit=-1.0) -> (coerced(x)=w1122:dbl)  [unwired: 1 out]
            n259 = In Range and Coerce(upper limit=0.0, x=w1108, lower limit=-1.0) -> (coerced(x)=w1112:dbl)  [unwired: 1 out]
            n260 = Select(t=w1122, s=w1103, f=w1116) -> (s? t:f=w1119:dbl)
            n261 = Wait (ms)(milliseconds to wait=u32 20) -> ()  [unwired: 1 out]
            n262 = Select(t=w1112, s=w1103, f=w1108) -> (s? t:f=w1109:dbl)
            n263 = call <vilib>:"CTRE_Phoenix_MotorControl_Set.vi"("error in (no error)"=w1123, "Output"=w1119, "Control Mode"=w1102, "PhoenixMotorControlDevRef"=w1124) -> ("error out"=w1117:errorcluster, "PhoenixMotorControlDevRef"=w1118:T6)  [unwired: 6 in]
            n264 = call <vilib>:"CTRE_Phoenix_MotorControl_Set.vi"("error in (no error)"=w1106, "Output"=w1109, "Control Mode"=w1102, "PhoenixMotorControlDevRef"=w1107) -> ("error out"=w1104:errorcluster, "PhoenixMotorControlDevRef"=w1105:T6)  [unwired: 6 in]
          }
          n265 = flat-sequence {
            tunnel: w1072 -> [w1086]
            tunnel: w1071 -> [w1085]
            tunnel: [w1084] -> w1070
            tunnel: [w1083] -> w1068
            tunnel: w1070 -> [w1100]
            tunnel: [w1099] -> w1069
            tunnel: w1068 -> [w1098]
            tunnel: [w1098] -> w1067
            frame #0 {
              n266 = while {
                shift-right: [w1095] -> w1084
                shift-left: w1085 -> [w1097]
                shift-right: [w1094] -> w1083
                shift-left: w1086 -> [w1096]
                stop <- w1093 stop-if-true
                w1092 = -0.6 ("Left axis value")
                # "Drive Back X Distance"
                n267 = call-poly <vilib>:"CTRE_Phoenix_MotorController_Get_TalonFX.vi"("PhoenixMotorControlDevRef"=w1096) -> ("PhoenixMotorControlDevRef"=w1094:T6, "Position (Raw Sensor Units)"=w1088:i32)  [unwired: 11 in, 2 out]
                n268 = call <vilib>:"WPI_RobotDriveTankDrive.vi"("Right axis value"=w1092, "Left axis value"=w1092, "RobotDriveDevRef"=w1097) -> ("RobotDriveDevRef"=w1095:T5)  [unwired: 6 in, 2 out]
                n269 = Divide(x=w1088, y=2048) -> (x/y=w1089:dbl)
                n270 = Round To Nearest(number=w1089) -> (nearest integer value=w1087:dbl)
                n271 = Less Or Equal?(x=w1087, y=-45) -> (x <= y?=w1093:bool)
                n272 = local write "Talon FX LEFT Moter Encoders"(w1087) -> ()
              }
            }
            frame #1 {
              w1101 = 0.0 ("Left axis value")
              n273 = call <vilib>:"WPI_RobotDriveTankDrive.vi"("Right axis value"=w1101, "Left axis value"=w1101, "RobotDriveDevRef"=w1100) -> ("RobotDriveDevRef"=w1099:T5)  [unwired: 6 in, 2 out]
            }
          }
        }
        frame #6 {
          n274 = call <vilib>:"CTRE_PigeonIMU_SetAccumZAngle.vi"("error in (no error)"=w1129, "Angle (Deg)"=0.0, "PigeonIMUDevRef"=w1128) -> ("error out"=w1126:errorcluster, "PigeonIMUDevRef"=w1127:T12)  [unwired: 7 in]
          n275 = Wait (ms)(milliseconds to wait=u32 250) -> ()  [unwired: 1 out]
        }
        frame #7 {
          w1148 = 0.0 ("Output")
          w1147 = T11 0 items=["PercentOutput"=0, "Position"=1, "Velocity"=2, "Current"=3, "Follower"=5, "MotionProfile"=6, "MotionMagic"=7, "MotionProfileArc"=10, "Disabled"=15] ("Control Mode")
          n276 = flat-sequence {
            tunnel: [w1156] -> w1143
            tunnel: w1140 -> [w1155]
            tunnel: w1141 -> [w1154]
            tunnel: w1142 -> [w1153]
            tunnel: w1143 -> [w1171]
            tunnel: [w1170] -> w1138
            frame #0 {
              # "Turn -15 degrees"
              n277 = while {
                shift-right: [w1167] -> w1156
                shift-left: w1155 -> [w1168]
                shift-right: [w1159] -> _
                shift-left: w1154 -> [w1161]
                tunnel: w1153 -> [w1160]
                tunnel: [w1158] -> _
                stop <- w1164 stop-if-true
                n278 = call-poly <vilib>:"CTRE_Phoenix_Pigeon2_GetStatus.vi"("error in (no error)"=w1161, "PigeonIMUDevRef"=w1160) -> ("error out"=w1159:errorcluster, "AccumGyro"=w1166:cluster{"X":dbl, "Y":dbl, "Z":dbl}, "PigeonIMUDevRef"=w1158:T12)  [unwired: 7 in]
                n279 = call-poly <vilib>:"WPI_RobotDriveArcadeDrive.vi"("Y axis value"=0.0, "X axis value"=0.4, "RobotDriveDevRef"=w1168) -> ("RobotDriveDevRef"=w1167:T5)  [unwired: 6 in, 2 out]
                n280 = Unbundle(w1166) -> ("Z"=w1157:dbl)  [unwired: 2 out]
                n281 = Less Or Equal?(x=w1157, y=-2.0) -> (x <= y?=w1164:bool)
                n282 = local write "Z"(w1157) -> ()
              }
            }
            frame #1 {
              w1169 = 0.0 ("Y axis value")
              # "Stop Turning"
              n283 = call-poly <vilib>:"WPI_RobotDriveArcadeDrive.vi"("Y axis value"=w1169, "X axis value"=w1169, "RobotDriveDevRef"=w1171) -> ("RobotDriveDevRef"=w1170:T5)  [unwired: 6 in, 2 out]
            }
          }
          n284 = call <vilib>:"CTRE_Phoenix_MotorControl_Set.vi"("error in (no error)"=w1151, "Output"=w1148, "Control Mode"=w1147, "PhoenixMotorControlDevRef"=w1152) -> ()  [unwired: 6 in, 2 out]
          n285 = call <vilib>:"CTRE_Phoenix_MotorControl_Set.vi"("error in (no error)"=w1149, "Output"=w1148, "Control Mode"=w1147, "PhoenixMotorControlDevRef"=w1150) -> ("error out"=w1144:errorcluster, "PhoenixMotorControlDevRef"=w1145:T6)  [unwired: 6 in]
        }
        frame #8 {
          n286 = call <vilib>:"CTRE_Phoenix_MotorControl_SetSelectedSensorPosition.vi"("New Sensor Position"=0, "PhoenixMotorControlDevRef"=w1173) -> ("PhoenixMotorControlDevRef"=w1174:T6)  [unwired: 8 in, 1 out]
        }
        frame #9 {
          # "Rev up shooter"
          n287 = flat-sequence {
            tunnel: [w1187] -> _
            tunnel: w1181 -> [w1189]
            tunnel: [w1188] -> w1183
            tunnel: w1182 -> [w1187]
            tunnel: w1183 -> [w1202]
            tunnel: [w1201] -> _
            frame #0 {
              n288 = while {
                shift-right: [w1198] -> w1188
                shift-left: w1189 -> [w1200]
                shift-right: [w1197] -> _
                shift-left: w1187 -> [w1199]
                stop <- w1196 stop-if-true
                w1195 = 0.5 ("Left axis value")
                # "Drive Back X Distance"
                n289 = call-poly <vilib>:"CTRE_Phoenix_MotorController_Get_TalonFX.vi"("PhoenixMotorControlDevRef"=w1199) -> ("PhoenixMotorControlDevRef"=w1197:T6, "Position (Raw Sensor Units)"=w1191:i32)  [unwired: 11 in, 2 out]
                n290 = call <vilib>:"WPI_RobotDriveTankDrive.vi"("Right axis value"=w1195, "Left axis value"=w1195, "RobotDriveDevRef"=w1200) -> ("RobotDriveDevRef"=w1198:T5)  [unwired: 6 in, 2 out]
                n291 = Divide(x=w1191, y=2048) -> (x/y=w1192:dbl)
                n292 = Round To Nearest(number=w1192) -> (nearest integer value=w1190:dbl)
                n293 = Greater Or Equal?(x=w1190, y=39) -> (x >= y?=w1196:bool)
                n294 = local write "Talon FX LEFT Moter Encoders"(w1190) -> ()
              }
            }
            frame #1 {
              w1203 = 0.0 ("Left axis value")
              n295 = call <vilib>:"WPI_RobotDriveTankDrive.vi"("Right axis value"=w1203, "Left axis value"=w1203, "RobotDriveDevRef"=w1202) -> ("RobotDriveDevRef"=w1201:T5)  [unwired: 6 in, 2 out]
            }
          }
          n296 = call <vilib>:"WPI_MotorControlSetOutput.vi"("Output"=0.4, "MotorControlDevRef"=w1186) -> ("MotorControlDevRef"=w1179:T6)  [unwired: 7 in, 2 out]
        }
        frame #10 {
          w1208 = T11 0 items=["PercentOutput"=0, "Position"=1, "Velocity"=2, "Current"=3, "Follower"=5, "MotionProfile"=6, "MotionMagic"=7, "MotionProfileArc"=10, "Disabled"=15] ("Control Mode")
          # "Index Note"
          # "Shoot"
          n297 = call <vilib>:"CTRE_Phoenix_MotorControl_Set.vi"("error in (no error)"=w1205, "Output"=0.5, "Control Mode"=w1208, "PhoenixMotorControlDevRef"=w1206) -> ("error out"=w1204:errorcluster, "PhoenixMotorControlDevRef"=w1207:T6)  [unwired: 6 in]
          n298 = Wait (ms)(milliseconds to wait=u32 1500) -> ()  [unwired: 1 out]
          n299 = call <vilib>:"WPI_MotorControlSetOutput.vi"("Output"=0.4, "MotorControlDevRef"=w1211) -> ("MotorControlDevRef"=w1210:T6)  [unwired: 7 in, 2 out]
        }
        frame #11 {
          w1216 = T11 0 items=["PercentOutput"=0, "Position"=1, "Velocity"=2, "Current"=3, "Follower"=5, "MotionProfile"=6, "MotionMagic"=7, "MotionProfileArc"=10, "Disabled"=15] ("Control Mode")
          # "Stop All Action"
          # "Index Note"
          n300 = call <vilib>:"CTRE_Phoenix_MotorControl_Set.vi"("error in (no error)"=w1217, "Output"=0.0, "Control Mode"=w1216, "PhoenixMotorControlDevRef"=w1218) -> ()  [unwired: 6 in, 2 out]
          n301 = call <vilib>:"WPI_MotorControlSetOutput.vi"("Output"=0.0, "MotorControlDevRef"=w1214) -> ()  [unwired: 7 in, 3 out]
        }
      }
    }
    frame "Left Position 3 Shoot 2" {
      n302 = call <vilib>:"WPI_MotorControlRefNum Registry Get.vi"("refnum name"="Shooter Motors") -> ("error out"=w1224:errorcluster, "MotorControlDevRef"=w1223:T6)  [unwired: 9 in]
      n303 = call <vilib>:"CTRE_PigeonIMU_RefNumRegistryGet.vi"("refnum name"="Robot Angle") -> ("error out"=w1220:errorcluster, "PigeonIMUDevRef"=w1221:T12)  [unwired: 9 in]
      n304 = call <vilib>:"WPI_RobotDriveRefNum Registry Get.vi"("refnum name"="Left and Right Motors") -> ("RobotDriveDevRef"=w1225:T5)  [unwired: 9 in, 1 out]
      n305 = call <vilib>:"CTRE_Phoenix_MotorControl_RefNumRegistryGet.vi"("refnum name"="Left Motors") -> ("error out"=w1227:errorcluster, "PhoenixMotorControlDevRef"=w1226:T6)  [unwired: 9 in]
      n306 = call <vilib>:"CTRE_Phoenix_MotorControl_RefNumRegistryGet.vi"("refnum name"="intake") -> ("error out"=w1229:errorcluster, "PhoenixMotorControlDevRef"=w1228:T6)  [unwired: 9 in]
      n307 = call <vilib>:"WPI_SwitchRefNum Registry Get.vi"("refnum name"="Intake Limit") -> ("error out"=w1232:errorcluster, "SwitchDevRef"=w1233:T14)  [unwired: 9 in]
      n308 = call <vilib>:"CTRE_Phoenix_MotorControl_RefNumRegistryGet.vi"("refnum name"="Indexer") -> ("error out"=w1230:errorcluster, "PhoenixMotorControlDevRef"=w1231:T6)  [unwired: 9 in]
      n309 = flat-sequence {
        tunnel: w1223 -> [w1360]
        tunnel: w1224 -> [w1359]
        tunnel: [w1356] -> w1333
        tunnel: [w1355] -> w1332
        tunnel: [w1354] -> w1331
        tunnel: [w1353] -> w1330
        tunnel: w1226 -> [w1347]
        tunnel: [w1349] -> w1329
        tunnel: w1227 -> [w1350]
        tunnel: [w1339] -> _
        tunnel: [w1339] -> w1328
        tunnel: [w1348] -> w1327
        tunnel: [w1341] -> _
        tunnel: [w1341] -> w1326
        tunnel: [w1340] -> _
        tunnel: [w1340] -> w1325
        tunnel: w1233 -> [w1345]
        tunnel: [w1345] -> w1324
        tunnel: w1232 -> [w1344]
        tunnel: [w1344] -> w1323
        tunnel: [w1342] -> _
        tunnel: w1230 -> [w1343]
        tunnel: w1231 -> [w1342]
        tunnel: w1229 -> [w1341]
        tunnel: w1228 -> [w1340]
        tunnel: w1225 -> [w1339]
        tunnel: w1221 -> [w1338]
        tunnel: w1220 -> [w1337]
        tunnel: [w1335] -> w1322
        tunnel: [w1334] -> w1321
        tunnel: w1333 -> [w1380]
        tunnel: w1332 -> [w1379]
        tunnel: [w1378] -> w1320
        tunnel: [w1377] -> w1319
        tunnel: w1331 -> [w1375]
        tunnel: w1330 -> [w1374]
        tunnel: [w1371] -> w1318
        tunnel: w1329 -> [w1370]
        tunnel: [w1370] -> w1317
        tunnel: [w1369] -> w1316
        tunnel: w1328 -> [w1369]
        tunnel: w1327 -> [w1371]
        tunnel: w1326 -> [w1368]
        tunnel: [w1368] -> w1315
        tunnel: w1325 -> [w1367]
        tunnel: [w1367] -> w1314
        tunnel: w1324 -> [w1366]
        tunnel: [w1366] -> w1313
        tunnel: w1323 -> [w1365]
        tunnel: [w1365] -> w1312
        tunnel: [w1364] -> w1311
        tunnel: [w1363] -> w1310
        tunnel: w1322 -> [w1362]
        tunnel: w1321 -> [w1361]
        tunnel: [w1362] -> w1309
        tunnel: [w1361] -> w1308
        tunnel: w1320 -> [w1403]
        tunnel: w1319 -> [w1402]
        tunnel: w1318 -> [w1400]
        tunnel: w1317 -> [w1399]
        tunnel: w1316 -> [w1398]
        tunnel: w1315 -> [w1384]
        tunnel: w1314 -> [w1385]
        tunnel: w1313 -> [w1390]
        tunnel: w1312 -> [w1389]
        tunnel: w1311 -> [w1396]
        tunnel: w1310 -> [w1395]
        tunnel: [w1397] -> w1307
        tunnel: [w1394] -> w1306
        tunnel: w1309 -> [w1394]
        tunnel: [w1393] -> w1305
        tunnel: w1308 -> [w1393]
        tunnel: [w1392] -> w1304
        tunnel: [w1391] -> w1303
        tunnel: [w1390] -> w1302
        tunnel: [w1389] -> w1301
        tunnel: [w1385] -> w1300
        tunnel: [w1384] -> w1299
        tunnel: [w1388] -> w1298
        tunnel: [w1387] -> w1297
        tunnel: [w1386] -> w1296
        tunnel: w1307 -> [w1431]
        tunnel: [w1421] -> w1295
        tunnel: [w1430] -> w1294
        tunnel: w1306 -> [w1429]
        tunnel: w1305 -> [w1428]
        tunnel: [w1427] -> w1293
        tunnel: w1304 -> [w1427]
        tunnel: [w1426] -> w1292
        tunnel: w1303 -> [w1426]
        tunnel: [w1425] -> w1291
        tunnel: w1302 -> [w1425]
        tunnel: w1301 -> [w1424]
        tunnel: [w1424] -> w1290
        tunnel: [w1423] -> w1289
        tunnel: w1300 -> [w1423]
        tunnel: w1299 -> [w1422]
        tunnel: [w1422] -> w1288
        tunnel: w1298 -> [w1421]
        tunnel: w1297 -> [_]
        tunnel: w1296 -> [w1416]
        tunnel: [w1419] -> w1287
        tunnel: [w1417] -> w1286
        tunnel: [w1416] -> w1285
        tunnel: w1295 -> [w1462]
        tunnel: [w1461] -> w1284
        tunnel: w1294 -> [w1459]
        tunnel: [w1459] -> w1283
        tunnel: w1293 -> [w1468]
        tunnel: [w1468] -> w1282
        tunnel: w1292 -> [w1467]
        tunnel: [w1467] -> w1281
        tunnel: w1291 -> [w1466]
        tunnel: [w1466] -> w1280
        tunnel: w1290 -> [w1465]
        tunnel: [w1465] -> w1279
        tunnel: w1289 -> [w1464]
        tunnel: [w1464] -> w1278
        tunnel: w1288 -> [w1463]
        tunnel: [w1463] -> w1277
        tunnel: w1287 -> [w1458]
        tunnel: [w1458] -> w1276
        tunnel: [w1457] -> w1275
        tunnel: w1286 -> [w1457]
        tunnel: [w1456] -> w1274
        tunnel: w1285 -> [w1456]
        tunnel: w1284 -> [w1477]
        tunnel: w1283 -> [w1476]
        tunnel: w1282 -> [w1482]
        tunnel: w1281 -> [w1483]
        tunnel: w1280 -> [w1485]
        tunnel: w1279 -> [w1484]
        tunnel: w1278 -> [w1487]
        tunnel: w1277 -> [w1486]
        tunnel: [w1481] -> w1273
        tunnel: [w1480] -> w1272
        tunnel: [w1478] -> w1271
        tunnel: [w1479] -> w1270
        tunnel: [w1474] -> w1269
        tunnel: [w1472] -> w1268
        tunnel: w1276 -> [w1471]
        tunnel: [w1471] -> w1267
        tunnel: w1275 -> [w1470]
        tunnel: [w1470] -> w1266
        tunnel: [w1469] -> w1265
        tunnel: w1274 -> [w1469]
        tunnel: w1273 -> [w1542]
        tunnel: [w1542] -> w1264
        tunnel: w1272 -> [w1541]
        tunnel: [w1541] -> w1263
        tunnel: w1271 -> [w1540]
        tunnel: [w1540] -> w1262
        tunnel: w1270 -> [w1539]
        tunnel: [w1539] -> w1261
        tunnel: w1269 -> [w1538]
        tunnel: [w1538] -> w1260
        tunnel: w1268 -> [w1537]
        tunnel: [w1537] -> w1259
        tunnel: w1267 -> [w1534]
        tunnel: w1266 -> [w1533]
        tunnel: w1265 -> [w1536]
        tunnel: [w1536] -> w1258
        tunnel: [w1532] -> w1257
        tunnel: [w1531] -> w1256
        tunnel: w1264 -> [w1557]
        tunnel: w1263 -> [w1556]
        tunnel: w1262 -> [w1555]
        tunnel: w1261 -> [w1554]
        tunnel: w1260 -> [w1545]
        tunnel: w1259 -> [w1544]
        tunnel: [w1551] -> w1255
        tunnel: w1258 -> [w1551]
        tunnel: [w1550] -> w1254
        tunnel: [w1549] -> w1253
        tunnel: w1257 -> [w1547]
        tunnel: w1256 -> [w1546]
        tunnel: [w1544] -> w1252
        tunnel: [w1543] -> w1251
        tunnel: w1255 -> [w1583]
        tunnel: [w1583] -> w1250
        tunnel: w1254 -> [w1582]
        tunnel: [w1582] -> w1249
        tunnel: w1253 -> [w1581]
        tunnel: [w1581] -> w1248
        tunnel: [w1579] -> w1247
        tunnel: w1252 -> [w1578]
        tunnel: w1251 -> [w1577]
        tunnel: [w1577] -> w1246
        tunnel: [w1584] -> w1243
        tunnel: w1250 -> [w1591]
        tunnel: [w1590] -> w1244
        tunnel: w1249 -> [w1590]
        tunnel: w1248 -> [w1589]
        tunnel: [w1589] -> w1245
        tunnel: w1247 -> [w1587]
        tunnel: w1246 -> [w1586]
        tunnel: [w1612] -> w1240
        tunnel: [w1609] -> w1241
        tunnel: w1245 -> [w1610]
        tunnel: w1244 -> [w1611]
        tunnel: w1243 -> [w1616]
        tunnel: [w1615] -> w1242
        tunnel: w1242 -> [w1619]
        tunnel: w1241 -> [w1622]
        tunnel: w1240 -> [w1623]
        frame #0 {
          w1351 = T11 0 items=["PercentOutput"=0, "Position"=1, "Velocity"=2, "Current"=3, "Follower"=5, "MotionProfile"=6, "MotionMagic"=7, "MotionProfileArc"=10, "Disabled"=15] ("Control Mode")
          # "Rev up Shooter"
          n310 = call <vilib>:"CTRE_PigeonIMU_SetAccumZAngle.vi"("error in (no error)"=w1337, "Angle (Deg)"=0.0, "PigeonIMUDevRef"=w1338) -> ("error out"=w1334:errorcluster, "PigeonIMUDevRef"=w1335:T12)  [unwired: 7 in]
          n311 = call <vilib>:"CTRE_Phoenix_MotorControl_SetSelectedSensorPosition.vi"("error in (no error)"=w1350, "New Sensor Position"=0, "PhoenixMotorControlDevRef"=w1347) -> ("error out"=w1349:errorcluster, "PhoenixMotorControlDevRef"=w1348:T6)  [unwired: 7 in]
          n312 = call <vilib>:"WPI_MotorControlSetOutput.vi"("error in (no error)"=w1359, "Output"=0.4, "MotorControlDevRef"=w1360) -> ("error out"=w1355:errorcluster, "MotorControlDevRef"=w1356:T6)  [unwired: 6 in, 1 out]
          n313 = Wait (ms)(milliseconds to wait=u32 750) -> ()  [unwired: 1 out]
          n314 = call <vilib>:"CTRE_Phoenix_MotorControl_Set.vi"("error in (no error)"=w1343, "Output"=0.0, "Control Mode"=w1351, "PhoenixMotorControlDevRef"=w1342) -> ("error out"=w1353:errorcluster, "PhoenixMotorControlDevRef"=w1354:T6)  [unwired: 6 in]
        }
        frame #1 {
          w1372 = T11 0 items=["PercentOutput"=0, "Position"=1, "Velocity"=2, "Current"=3, "Follower"=5, "MotionProfile"=6, "MotionMagic"=7, "MotionProfileArc"=10, "Disabled"=15] ("Control Mode")
          # "Index and then Shoot"
          n315 = Wait (ms)(milliseconds to wait=u32 1500) -> ()  [unwired: 1 out]
          n316 = call <vilib>:"WPI_MotorControlSetOutput.vi"("error in (no error)"=w1379, "Output"=0.4, "MotorControlDevRef"=w1380) -> ("error out"=w1377:errorcluster, "MotorControlDevRef"=w1378:T6)  [unwired: 6 in, 1 out]
          n317 = call <vilib>:"CTRE_Phoenix_MotorControl_Set.vi"("error in (no error)"=w1374, "Output"=0.4, "Control Mode"=w1372, "PhoenixMotorControlDevRef"=w1375) -> ("error out"=w1363:errorcluster, "PhoenixMotorControlDevRef"=w1364:T6)  [unwired: 6 in]
        }
        frame #2 {
          w1383 = T11 0 items=["PercentOutput"=0, "Position"=1, "Velocity"=2, "Current"=3, "Follower"=5, "MotionProfile"=6, "MotionMagic"=7, "MotionProfileArc"=10, "Disabled"=15] ("Control Mode")
          # "Stop Indexing/intaking"
          # "3)Stop index and shooter and drive back a little"
          n318 = call <vilib>:"CTRE_Phoenix_MotorControl_Set.vi"("error in (no error)"=w1395, "Output"=0.0, "Control Mode"=w1383, "PhoenixMotorControlDevRef"=w1396) -> ("error out"=w1392:errorcluster, "PhoenixMotorControlDevRef"=w1391:T6)  [unwired: 6 in]
          n319 = while {
            shift-right: [w1413] -> w1397
            shift-left: w1398 -> [w1415]
            shift-right: [w1412] -> w1388
            shift-left: w1400 -> [w1414]
            tunnel: w1399 -> [w1405]
            stop <- w1411 stop-if-true
            w1410 = -0.4 ("Left axis value")
            # "Drive Back X Distance"
            n320 = call-poly <vilib>:"CTRE_Phoenix_MotorController_Get_TalonFX.vi"("PhoenixMotorControlDevRef"=w1414, "error in"=w1405) -> ("PhoenixMotorControlDevRef"=w1412:T6, "Position (Raw Sensor Units)"=w1406:i32)  [unwired: 10 in, 2 out]
            n321 = call <vilib>:"WPI_RobotDriveTankDrive.vi"("Right axis value"=w1410, "Left axis value"=w1410, "RobotDriveDevRef"=w1415) -> ("RobotDriveDevRef"=w1413:T5)  [unwired: 6 in, 2 out]
            n322 = Divide(x=w1406, y=2048) -> (x/y=w1407:dbl)
            n323 = Round To Nearest(number=w1407) -> (nearest integer value=w1404:dbl)
            n324 = Less Or Equal?(x=w1404, y=-12) -> (x <= y?=w1411:bool)
            n325 = local write "Talon FX LEFT Moter Encoders"(w1404) -> ()
          }
          n326 = call <vilib>:"WPI_MotorControlSetOutput.vi"("error in (no error)"=w1402, "Output"=0.0, "MotorControlDevRef"=w1403) -> ("error out"=w1387:errorcluster, "MotorControlDevRef"=w1386:T6)  [unwired: 6 in, 1 out]
        }
        frame #3 {
          # "Turn X Degrees"
          n327 = flat-sequence {
            tunnel: [w1438] -> w1432
            tunnel: w1431 -> [w1437]
            tunnel: w1429 -> [w1436]
            tunnel: w1428 -> [w1435]
            tunnel: [w1434] -> w1420
            tunnel: [w1433] -> w1418
            tunnel: w1432 -> [w1455]
            tunnel: [w1454] -> w1430
            tunnel: w1420 -> [w1451]
            tunnel: [w1452] -> w1419
            tunnel: w1418 -> [w1452]
            tunnel: [w1451] -> w1417
            frame #0 {
              # "Turn -45 degrees"
              n328 = while {
                shift-right: [w1449] -> w1438
                shift-left: w1437 -> [w1450]
                shift-right: [w1442] -> w1434
                shift-left: w1436 -> [w1448]
                tunnel: w1435 -> [w1441]
                tunnel: [w1440] -> w1433
                stop <- w1445 stop-if-true
                n329 = call-poly <vilib>:"CTRE_Phoenix_Pigeon2_GetStatus.vi"("error in (no error)"=w1441, "PigeonIMUDevRef"=w1448) -> ("error out"=w1440:errorcluster, "AccumGyro"=w1447:cluster{"X":dbl, "Y":dbl, "Z":dbl}, "PigeonIMUDevRef"=w1442:T12)  [unwired: 7 in]
                n330 = call-poly <vilib>:"WPI_RobotDriveArcadeDrive.vi"("Y axis value"=0.0, "X axis value"=0.4, "RobotDriveDevRef"=w1450) -> ("RobotDriveDevRef"=w1449:T5)  [unwired: 6 in, 2 out]
                n331 = Unbundle(w1447) -> ("Z"=w1439:dbl)  [unwired: 2 out]
                n332 = Less Or Equal?(x=w1439, y=-23.0) -> (x <= y?=w1445:bool)
                n333 = local write "Z"(w1439) -> ()
              }
            }
            frame #1 {
              w1453 = 0.0 ("Y axis value")
              # "Stop Turning"
              n334 = call-poly <vilib>:"WPI_RobotDriveArcadeDrive.vi"("Y axis value"=w1453, "X axis value"=w1453, "RobotDriveDevRef"=w1455) -> ("RobotDriveDevRef"=w1454:T5)  [unwired: 6 in, 2 out]
            }
          }
        }
        frame #4 {
          n335 = call <vilib>:"CTRE_Phoenix_MotorControl_SetSelectedSensorPosition.vi"("New Sensor Position"=0, "PhoenixMotorControlDevRef"=w1462) -> ("PhoenixMotorControlDevRef"=w1461:T6)  [unwired: 8 in, 1 out]
        }
        frame #5 {
          # "5)Drive x distance and run indexer/intake"
          n336 = while {
            shift-right: [w1524] -> w1481
            shift-left: w1487 -> [w1530]
            shift-right: [w1523] -> w1480
            shift-left: w1486 -> [w1529]
            tunnel: w1485 -> [w1520]
            tunnel: w1484 -> [w1519]
            tunnel: w1483 -> [w1513]
            tunnel: w1482 -> [w1512]
            tunnel: [w1511] -> w1478
            tunnel: [w1510] -> w1479
            stop <- w1509 stop-if-true
            w1514 = 0.5 ("x")
            w1522 = 1.0 ("x")
            w1508 = T11 0 items=["PercentOutput"=0, "Position"=1, "Velocity"=2, "Current"=3, "Follower"=5, "MotionProfile"=6, "MotionMagic"=7, "MotionProfileArc"=10, "Disabled"=15] ("Control Mode")
            n337 = call <vilib>:"WPI_SwitchGetLimitValue.vi"("error in (no error)"=w1519, "SwitchDevRef"=w1520) -> ("Switch Pressed"=w1509:bool)  [unwired: 7 in, 2 out]
            n338 = local write "Limit Switch"(w1509) -> ()
            n339 = In Range and Coerce(upper limit=0.0, x=w1522, lower limit=-1.0) -> (coerced(x)=w1528:dbl)  [unwired: 1 out]
            n340 = In Range and Coerce(upper limit=0.0, x=w1514, lower limit=-1.0) -> (coerced(x)=w1518:dbl)  [unwired: 1 out]
            n341 = Select(t=w1528, s=w1509, f=w1522) -> (s? t:f=w1525:dbl)
            n342 = Wait (ms)(milliseconds to wait=u32 20) -> ()  [unwired: 1 out]
            n343 = Select(t=w1518, s=w1509, f=w1514) -> (s? t:f=w1515:dbl)
            n344 = call <vilib>:"CTRE_Phoenix_MotorControl_Set.vi"("error in (no error)"=w1529, "Output"=w1525, "Control Mode"=w1508, "PhoenixMotorControlDevRef"=w1530) -> ("error out"=w1523:errorcluster, "PhoenixMotorControlDevRef"=w1524:T6)  [unwired: 6 in]
            n345 = call <vilib>:"CTRE_Phoenix_MotorControl_Set.vi"("error in (no error)"=w1512, "Output"=w1515, "Control Mode"=w1508, "PhoenixMotorControlDevRef"=w1513) -> ("error out"=w1510:errorcluster, "PhoenixMotorControlDevRef"=w1511:T6)  [unwired: 6 in]
          }
          n346 = flat-sequence {
            tunnel: w1477 -> [w1491]
            tunnel: w1476 -> [w1490]
            tunnel: [w1489] -> w1475
            tunnel: [w1488] -> w1473
            tunnel: w1475 -> [w1506]
            tunnel: [w1505] -> w1474
            tunnel: w1473 -> [w1504]
            tunnel: [w1504] -> w1472
            frame #0 {
              n347 = while {
                shift-right: [w1501] -> w1489
                shift-left: w1490 -> [w1503]
                shift-right: [w1500] -> w1488
                shift-left: w1491 -> [w1502]
                stop <- w1499 stop-if-true
                w1498 = -0.6 ("Left axis value")
                # "Drive Back X Distance"
                n348 = call-poly <vilib>:"CTRE_Phoenix_MotorController_Get_TalonFX.vi"("PhoenixMotorControlDevRef"=w1502) -> ("PhoenixMotorControlDevRef"=w1500:T6, "Position (Raw Sensor Units)"=w1494:i32)  [unwired: 11 in, 2 out]
                n349 = call <vilib>:"WPI_RobotDriveTankDrive.vi"("Right axis value"=w1498, "Left axis value"=w1498, "RobotDriveDevRef"=w1503) -> ("RobotDriveDevRef"=w1501:T5)  [unwired: 6 in, 2 out]
                n350 = Divide(x=w1494, y=2048) -> (x/y=w1495:dbl)
                n351 = Round To Nearest(number=w1495) -> (nearest integer value=w1493:dbl)
                n352 = Less Or Equal?(x=w1493, y=-45) -> (x <= y?=w1499:bool)
                n353 = local write "Talon FX LEFT Moter Encoders"(w1493) -> ()
                n354 = Wait (ms)(milliseconds to wait=u32 100) -> ()  [unwired: 1 out]
              }
            }
            frame #1 {
              w1507 = 0.0 ("Left axis value")
              n355 = call <vilib>:"WPI_RobotDriveTankDrive.vi"("Right axis value"=w1507, "Left axis value"=w1507, "RobotDriveDevRef"=w1506) -> ("RobotDriveDevRef"=w1505:T5)  [unwired: 6 in, 2 out]
            }
          }
        }
        frame #6 {
          n356 = call <vilib>:"CTRE_PigeonIMU_SetAccumZAngle.vi"("error in (no error)"=w1534, "Angle (Deg)"=0.0, "PigeonIMUDevRef"=w1533) -> ("error out"=w1531:errorcluster, "PigeonIMUDevRef"=w1532:T12)  [unwired: 7 in]
        }
        frame #7 {
          w1553 = 0.0 ("Output")
          w1552 = T11 0 items=["PercentOutput"=0, "Position"=1, "Velocity"=2, "Current"=3, "Follower"=5, "MotionProfile"=6, "MotionMagic"=7, "MotionProfileArc"=10, "Disabled"=15] ("Control Mode")
          n357 = flat-sequence {
            tunnel: [w1561] -> w1548
            tunnel: w1545 -> [w1560]
            tunnel: w1546 -> [w1559]
            tunnel: w1547 -> [w1558]
            tunnel: w1548 -> [w1576]
            tunnel: [w1575] -> w1543
            frame #0 {
              # "Turn -15 degrees"
              n358 = while {
                shift-right: [w1572] -> w1561
                shift-left: w1560 -> [w1573]
                shift-right: [w1564] -> _
                shift-left: w1559 -> [w1566]
                tunnel: w1558 -> [w1565]
                tunnel: [w1563] -> _
                stop <- w1569 stop-if-true
                n359 = call-poly <vilib>:"CTRE_Phoenix_Pigeon2_GetStatus.vi"("error in (no error)"=w1566, "PigeonIMUDevRef"=w1565) -> ("error out"=w1564:errorcluster, "AccumGyro"=w1571:cluster{"X":dbl, "Y":dbl, "Z":dbl}, "PigeonIMUDevRef"=w1563:T12)  [unwired: 7 in]
                n360 = call-poly <vilib>:"WPI_RobotDriveArcadeDrive.vi"("Y axis value"=0.0, "X axis value"=-0.4, "RobotDriveDevRef"=w1573) -> ("RobotDriveDevRef"=w1572:T5)  [unwired: 6 in, 2 out]
                n361 = Unbundle(w1571) -> ("Z"=w1562:dbl)  [unwired: 2 out]
                n362 = Greater Or Equal?(x=w1562, y=5.0) -> (x >= y?=w1569:bool)
                n363 = local write "Z"(w1562) -> ()
              }
            }
            frame #1 {
              w1574 = 0.0 ("Y axis value")
              # "Stop Turning"
              n364 = call-poly <vilib>:"WPI_RobotDriveArcadeDrive.vi"("Y axis value"=w1574, "X axis value"=w1574, "RobotDriveDevRef"=w1576) -> ("RobotDriveDevRef"=w1575:T5)  [unwired: 6 in, 2 out]
            }
          }
          n365 = call <vilib>:"CTRE_Phoenix_MotorControl_Set.vi"("error in (no error)"=w1556, "Output"=w1553, "Control Mode"=w1552, "PhoenixMotorControlDevRef"=w1557) -> ()  [unwired: 6 in, 2 out]
          n366 = call <vilib>:"CTRE_Phoenix_MotorControl_Set.vi"("error in (no error)"=w1554, "Output"=w1553, "Control Mode"=w1552, "PhoenixMotorControlDevRef"=w1555) -> ("error out"=w1549:errorcluster, "PhoenixMotorControlDevRef"=w1550:T6)  [unwired: 6 in]
        }
        frame #8 {
          n367 = call <vilib>:"CTRE_Phoenix_MotorControl_SetSelectedSensorPosition.vi"("New Sensor Position"=0, "PhoenixMotorControlDevRef"=w1578) -> ("PhoenixMotorControlDevRef"=w1579:T6)  [unwired: 8 in, 1 out]
        }
        frame #9 {
          # "Rev up shooter"
          n368 = flat-sequence {
            tunnel: [w1592] -> _
            tunnel: w1586 -> [w1594]
            tunnel: [w1593] -> w1588
            tunnel: w1587 -> [w1592]
            tunnel: w1588 -> [w1607]
            tunnel: [w1606] -> _
            frame #0 {
              n369 = while {
                shift-right: [w1603] -> w1593
                shift-left: w1594 -> [w1605]
                shift-right: [w1602] -> _
                shift-left: w1592 -> [w1604]
                stop <- w1601 stop-if-true
                w1600 = 0.5 ("Left axis value")
                # "Drive Back X Distance"
                n370 = call-poly <vilib>:"CTRE_Phoenix_MotorController_Get_TalonFX.vi"("PhoenixMotorControlDevRef"=w1604) -> ("PhoenixMotorControlDevRef"=w1602:T6, "Position (Raw Sensor Units)"=w1596:i32)  [unwired: 11 in, 2 out]
                n371 = call <vilib>:"WPI_RobotDriveTankDrive.vi"("Right axis value"=w1600, "Left axis value"=w1600, "RobotDriveDevRef"=w1605) -> ("RobotDriveDevRef"=w1603:T5)  [unwired: 6 in, 2 out]
                n372 = Divide(x=w1596, y=2048) -> (x/y=w1597:dbl)
                n373 = Round To Nearest(number=w1597) -> (nearest integer value=w1595:dbl)
                n374 = Greater Or Equal?(x=w1595, y=54) -> (x >= y?=w1601:bool)
                n375 = local write "Talon FX LEFT Moter Encoders"(w1595) -> ()
              }
            }
            frame #1 {
              w1608 = 0.0 ("Left axis value")
              n376 = call <vilib>:"WPI_RobotDriveTankDrive.vi"("Right axis value"=w1608, "Left axis value"=w1608, "RobotDriveDevRef"=w1607) -> ("RobotDriveDevRef"=w1606:T5)  [unwired: 6 in, 2 out]
            }
          }
          n377 = call <vilib>:"WPI_MotorControlSetOutput.vi"("Output"=0.4, "MotorControlDevRef"=w1591) -> ("MotorControlDevRef"=w1584:T6)  [unwired: 7 in, 2 out]
        }
        frame #10 {
          w1613 = T11 0 items=["PercentOutput"=0, "Position"=1, "Velocity"=2, "Current"=3, "Follower"=5, "MotionProfile"=6, "MotionMagic"=7, "MotionProfileArc"=10, "Disabled"=15] ("Control Mode")
          # "Index Note"
          # "Shoot"
          n378 = call <vilib>:"CTRE_Phoenix_MotorControl_Set.vi"("error in (no error)"=w1610, "Output"=0.5, "Control Mode"=w1613, "PhoenixMotorControlDevRef"=w1611) -> ("error out"=w1609:errorcluster, "PhoenixMotorControlDevRef"=w1612:T6)  [unwired: 6 in]
          n379 = Wait (ms)(milliseconds to wait=u32 1500) -> ()  [unwired: 1 out]
          n380 = call <vilib>:"WPI_MotorControlSetOutput.vi"("Output"=0.4, "MotorControlDevRef"=w1616) -> ("MotorControlDevRef"=w1615:T6)  [unwired: 7 in, 2 out]
        }
        frame #11 {
          w1621 = T11 0 items=["PercentOutput"=0, "Position"=1, "Velocity"=2, "Current"=3, "Follower"=5, "MotionProfile"=6, "MotionMagic"=7, "MotionProfileArc"=10, "Disabled"=15] ("Control Mode")
          # "Stop All Action"
          # "Index Note"
          n381 = call <vilib>:"CTRE_Phoenix_MotorControl_Set.vi"("error in (no error)"=w1622, "Output"=0.0, "Control Mode"=w1621, "PhoenixMotorControlDevRef"=w1623) -> ()  [unwired: 6 in, 2 out]
          n382 = call <vilib>:"WPI_MotorControlSetOutput.vi"("Output"=0.0, "MotorControlDevRef"=w1619) -> ()  [unwired: 7 in, 3 out]
        }
      }
    }
    frame "Your Turn" {
    }
  }
